vi "ゲージデータリセット.vi"(8 "測定周期/ms":dbl) -> (11 "実測設定項目配列_\nメインからの転記":T1[](array[typedef]) {"測定モード" items=["単発測定モード", "連続測定モード", "多点測定モード"]})   [LabVIEW 2021]
uses:
  <vilib>/Utility/config.llb/Read Key (U32).vi
  <vilib>/Utility/config.llb/Read Key (String).vi
  <vilib>/Utility/config.llb/Read Key (I32).vi
  <vilib>/Utility/config.llb/Read Key (Boolean).vi
  <vilib>/Utility/config.llb/NI_LVConfig.lvlib
panel:
  out "メイン設定_設定 12":T1 {"測定モード" items=["単発測定モード", "連続測定モード", "多点測定モード"]}
  out "メイン設定_設定 11":T1 {"測定モード" items=["単発測定モード", "連続測定モード", "多点測定モード"]}
  out "メイン設定_設定 10":T1 {"測定モード" items=["単発測定モード", "連続測定モード", "多点測定モード"]}
  out "メイン設定_設定 9":T1 {"測定モード" items=["単発測定モード", "連続測定モード", "多点測定モード"]}
  out "メイン設定_設定 8":T1 {"測定モード" items=["単発測定モード", "連続測定モード", "多点測定モード"]}
  out "メイン設定_設定 7":T1 {"測定モード" items=["単発測定モード", "連続測定モード", "多点測定モード"]}
  out "メイン設定_設定 6":T1 {"測定モード" items=["単発測定モード", "連続測定モード", "多点測定モード"]}
  out "メイン設定_設定 5":T1 {"測定モード" items=["単発測定モード", "連続測定モード", "多点測定モード"]}
  out "メイン設定_設定 4":T1 {"測定モード" items=["単発測定モード", "連続測定モード", "多点測定モード"]}
  out "メイン設定_設定 3":T1 {"測定モード" items=["単発測定モード", "連続測定モード", "多点測定モード"]}
  out "メイン設定_設定 2":T1 {"測定モード" items=["単発測定モード", "連続測定モード", "多点測定モード"]}
  out "メイン設定_設定 1":T1 {"測定モード" items=["単発測定モード", "連続測定モード", "多点測定モード"]}
  out "setup.iniエラーout":errorcluster caption="エラー入力（エラーなし）"
  out "iniフォルダパス取得":path
  in  "setup.iniエラーin":errorcluster caption="エラー入力（エラーなし）"
  out "ゲージエラー 12":errorcluster caption="エラー入力 (エラーなし)"
  out "ゲージエラー 11":errorcluster caption="エラー入力 (エラーなし)"
  out "ゲージエラー 10":errorcluster caption="エラー入力 (エラーなし)"
  out "ゲージエラー 9":errorcluster caption="エラー入力 (エラーなし)"
  out "ゲージエラー 8":errorcluster caption="エラー入力 (エラーなし)"
  out "ゲージエラー 7":errorcluster caption="エラー入力 (エラーなし)"
  out "ゲージエラー 6":errorcluster caption="エラー入力 (エラーなし)"
  out "ゲージエラー 5":errorcluster caption="エラー入力 (エラーなし)"
  out "ゲージエラー 4":errorcluster caption="エラー入力 (エラーなし)"
  out "ゲージエラー 3":errorcluster caption="エラー入力 (エラーなし)"
  out "ゲージエラー 2":errorcluster caption="エラー入力 (エラーなし)"
  out "ゲージエラー 1":errorcluster caption="エラー入力 (エラーなし)"
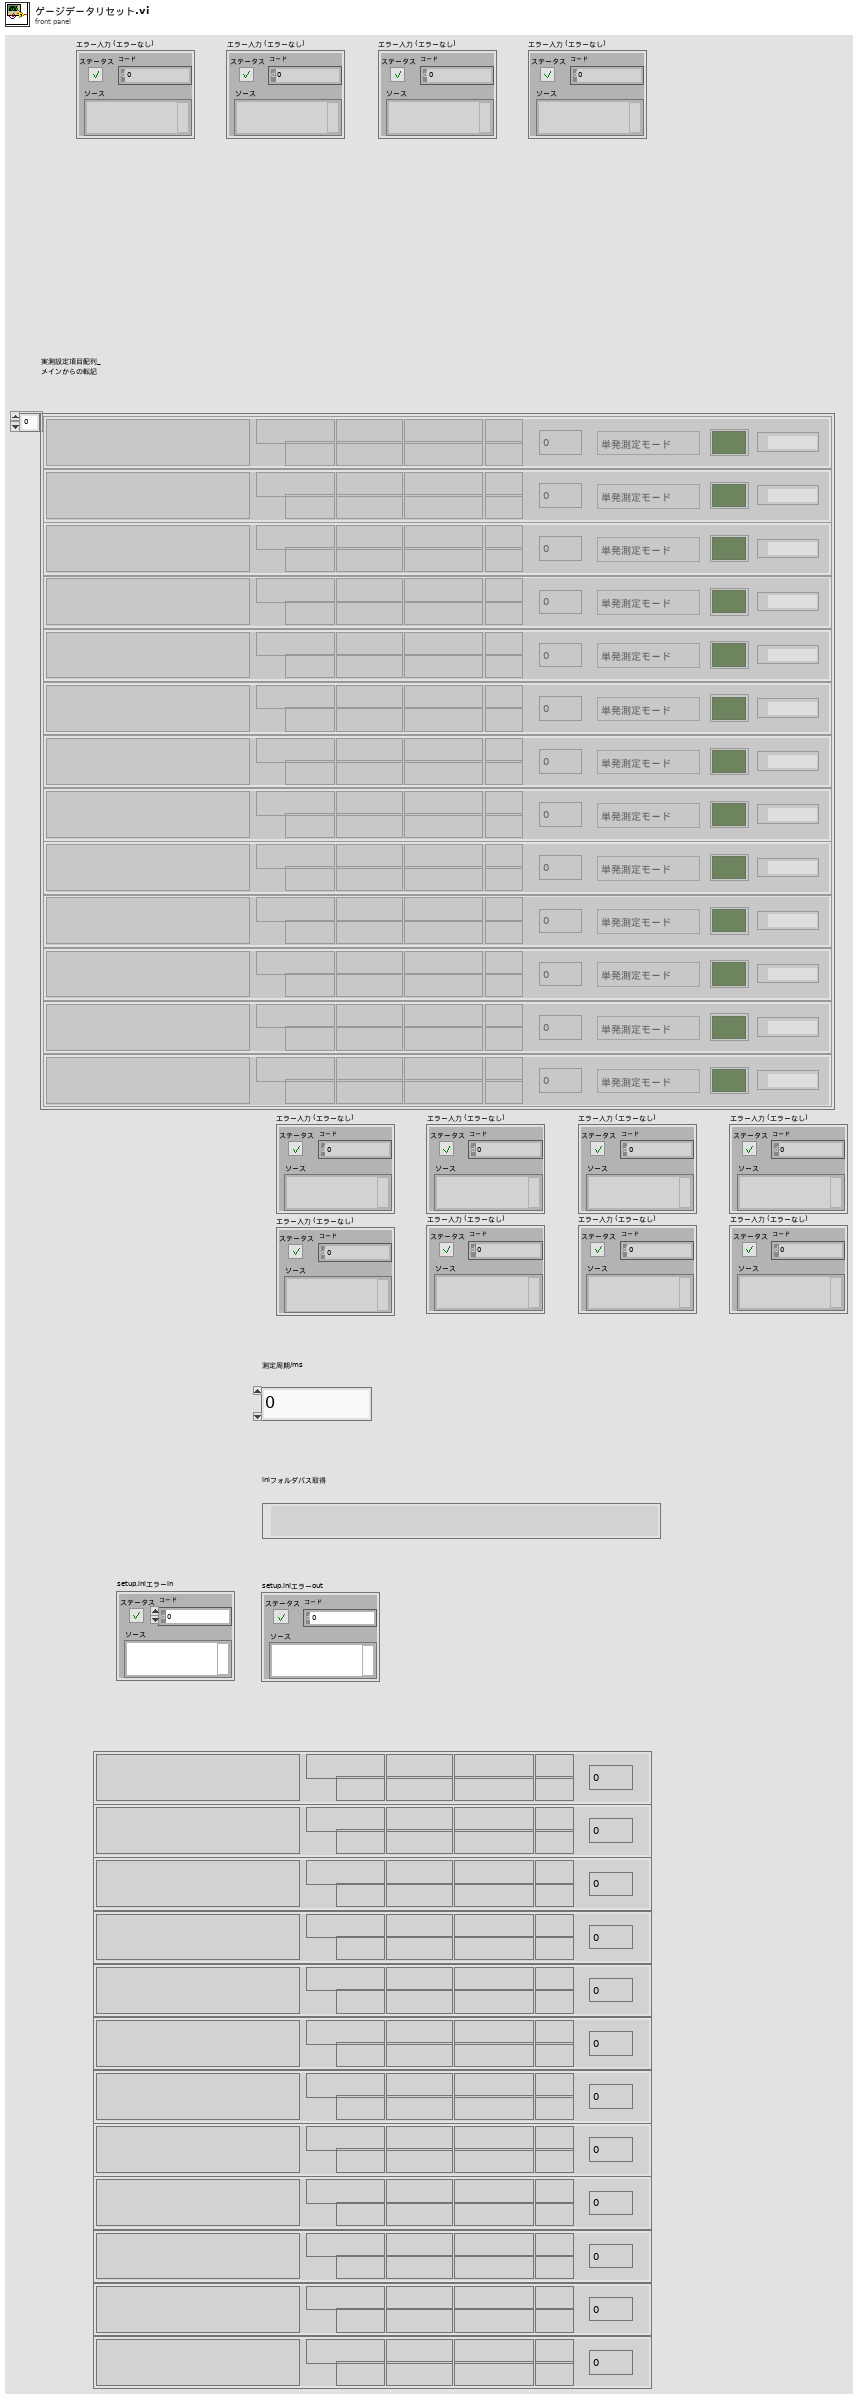
[diagram p1: front panel]
types:
  T1 = typedef "設定全項目制御器.ctl" = cluster{"規格":string, "規格上限":string, "規格下限":string, "ポートNo.":dbl, "測定モード":u16, "規格単位":string, "品質チェック項目":string, "測定周期":dbl, "実測値MAX":string, "実測値MIN":string, "実測値(MAX)":string, "実測値(MIN)":string, "測定画面表示ボタン":bool, "ゲージポートNo":refnum<visa-resource-name>}
  T2 = typedef "NI_LVConfig.lvlib/Config Data RefNum.ctl" = refnum<k1>
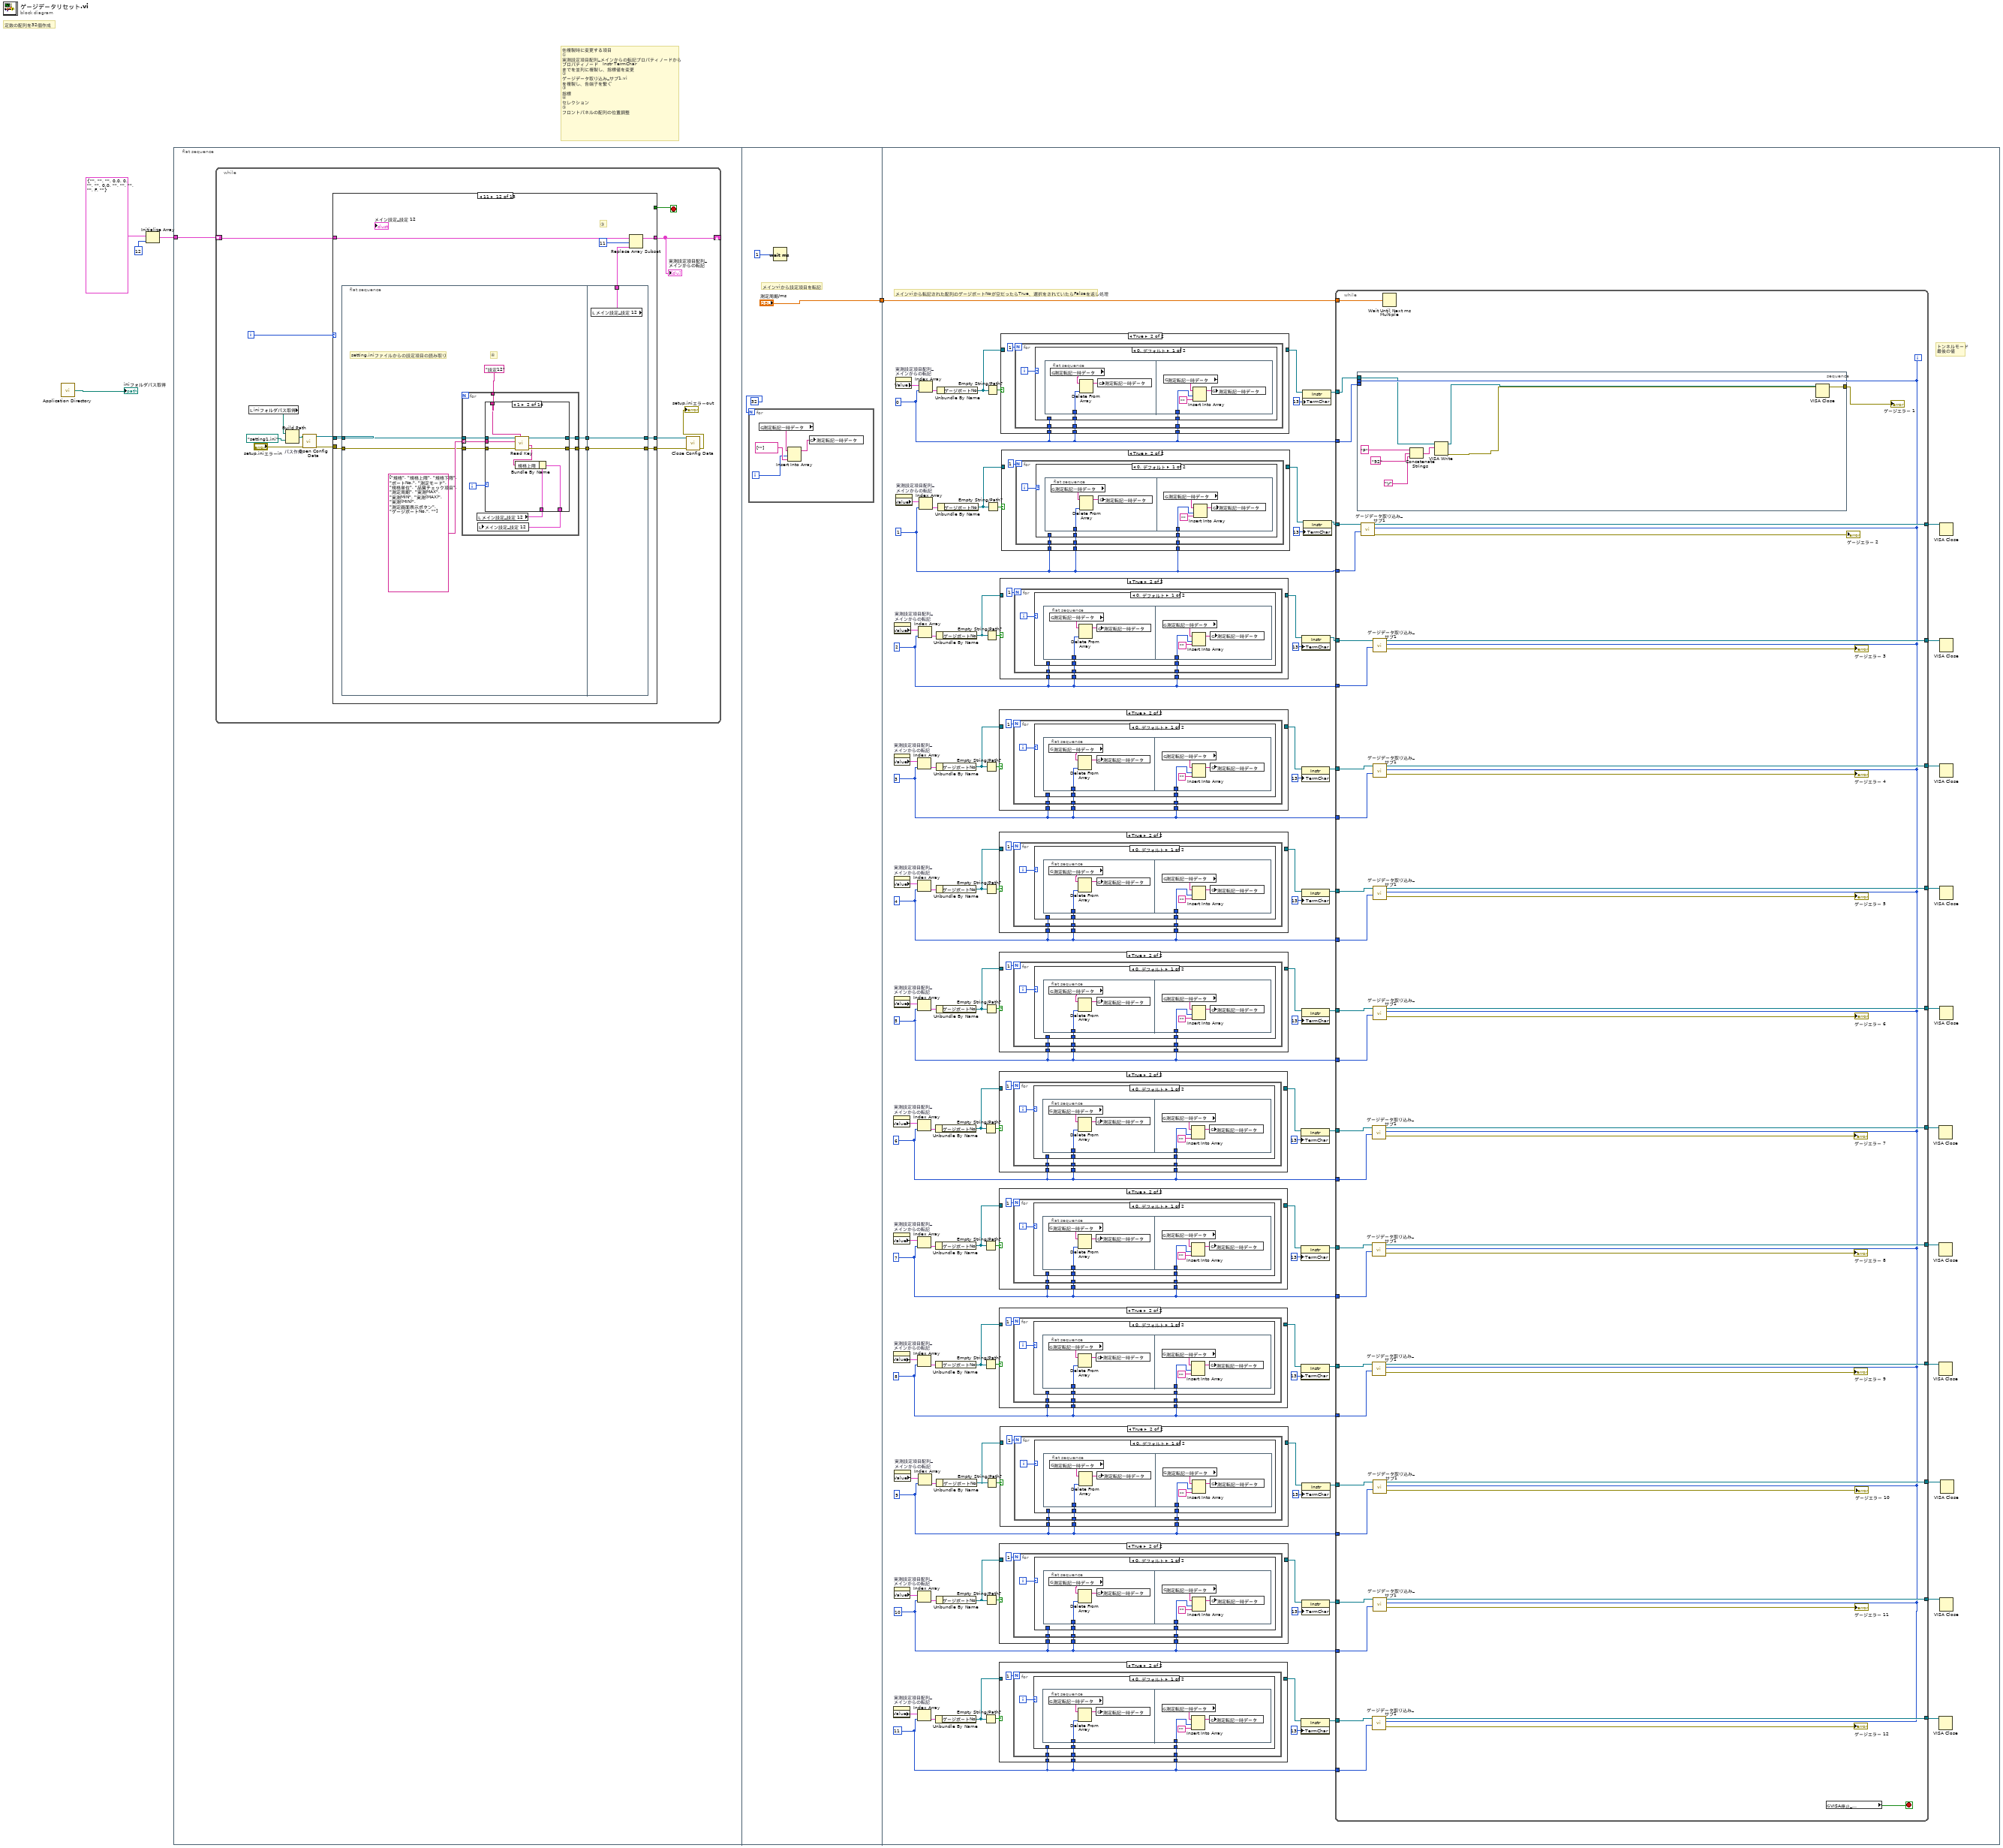
[diagram p0: block diagram]
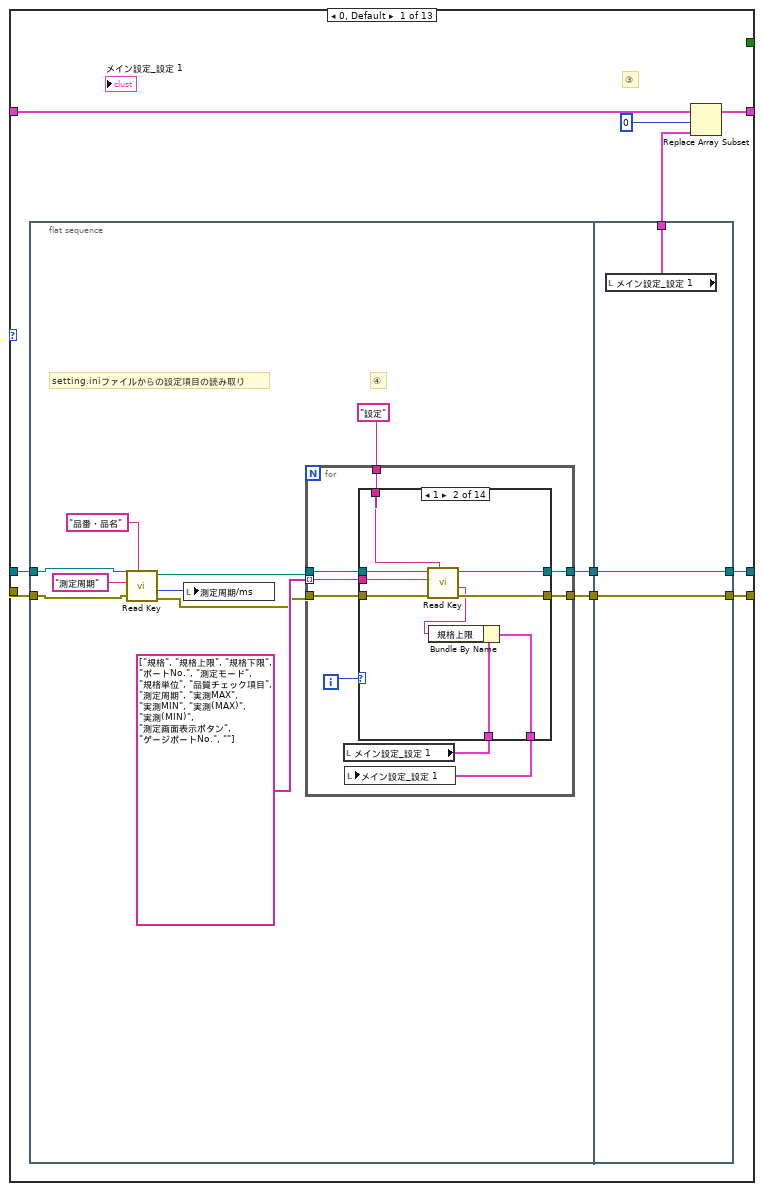
[diagram p2: hidden frame]
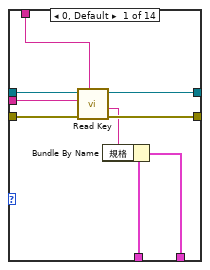
[diagram p3: hidden frame]
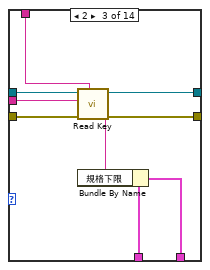
[diagram p4: hidden frame]
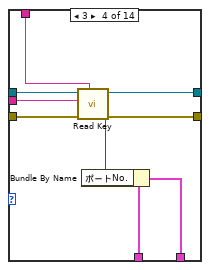
[diagram p5: hidden frame]
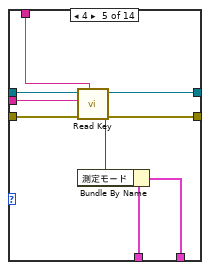
[diagram p6: hidden frame]
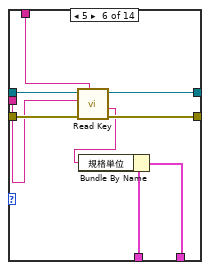
[diagram p7: hidden frame]
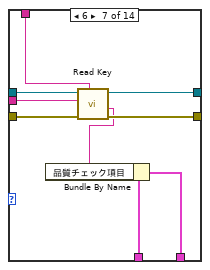
[diagram p8: hidden frame]
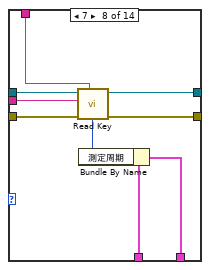
[diagram p9: hidden frame]
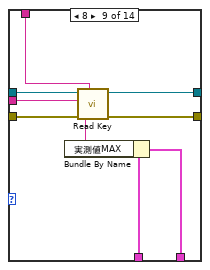
[diagram p10: hidden frame]
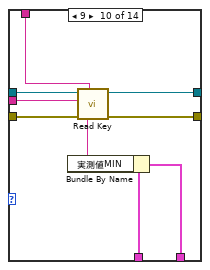
[diagram p11: hidden frame]
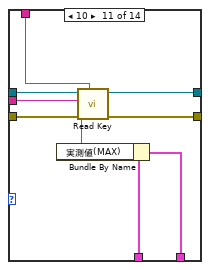
[diagram p12: hidden frame]
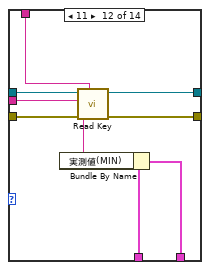
[diagram p13: hidden frame]
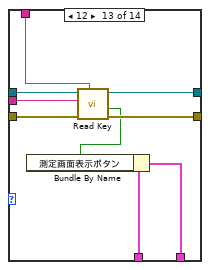
[diagram p14: hidden frame]
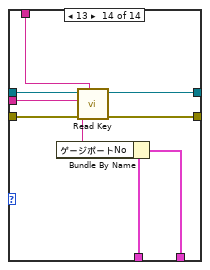
[diagram p15: hidden frame]
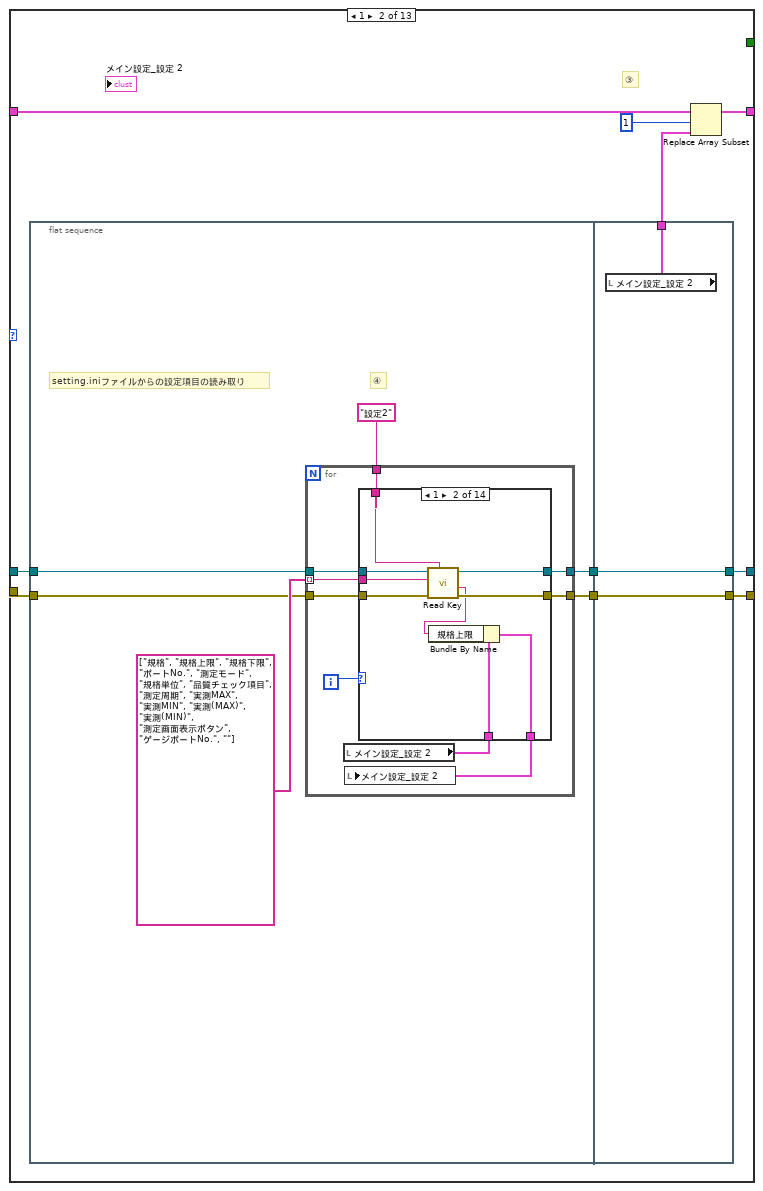
[diagram p16: hidden frame]
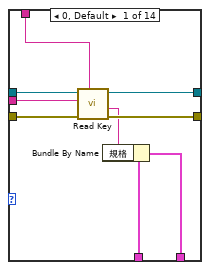
[diagram p17: hidden frame]
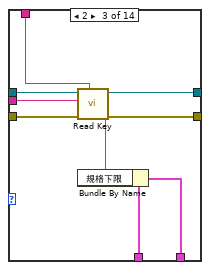
[diagram p18: hidden frame]
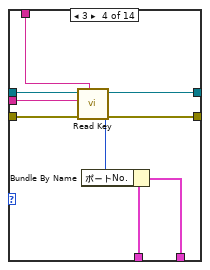
[diagram p19: hidden frame]
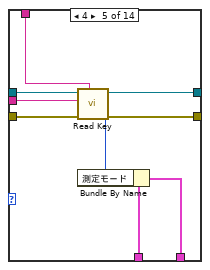
[diagram p20: hidden frame]
diagram:
  # "他複製時に変更する項目\n①\n実測設定項目配列_メインからの転記プロパティノードから\nプロパティノード　Instr TermChar\nまでを並列に複製し、指標値を変更\n②\nゲージデータ取り込み_サブ1.vi\nを複製し、各端子を繋ぐ\n③\n指標\n④\nセレクション\n⑤\nフロントパネルの配列の位置調整"
  # "定数の配列を32個作成"
  n1 = call <vilib>:"Application Directory.vi"() -> ("Application Directory"=→"iniフォルダパス取得":path)
  n2 = Initialize Array(T1 {"規格"="", "規格上限"="", "規格下限"="", "ポートNo."=0.0, "測定モード"=0, "規格単位"="", "品質チェック項目"="", "測定周期"=0.0, "実測値MAX"="", "実測値MIN"="", "実測値(MAX)"="", "実測値(MIN)"="", "測定画面表示ボタン"=FALSE, "ゲージポートNo"=""} ("メイン設定_設定"), 12) -> (w1:T1[])
  n3 = flat-sequence {
    tunnel: w1 -> [w6]
    tunnel: ["測定周期/ms"] -> w5
    tunnel: w5 -> [w1982]
    frame #0 {
      n4 = while {
        shift-right: [w7] -> _
        shift-left: w6 -> [w9]
        i -> [w14]
        stop <- w8 stop-if-true
        n5 = local read "iniフォルダパス取得"() -> (w19:path)
        n6 = Build Path "パス作成"(base path=w19, name or relative path=path "setting1.ini") -> (appended path=w18:path)
        n7 = call <vilib>:"Open Config Data.vi"("error in (no error)"="setup.iniエラーin", "configuration file path"=w18) -> ("error out"=w12:errorcluster, "refnum"=w13:T2)  [unwired: 1 in, 7 out]
        n8 = case shown="11" w14 {
          tunnel: w13 -> [w29 w188 w342 w496 w650 w804 w958 w1112 w1266 w1420 w1574 w1728 w1874]
          tunnel: w12 -> [w28 w187 w341 w495 w649 w803 w957 w1111 w1265 w1419 w1573 w1727 w1873]
          tunnel: [w27 w186 w340 w494 w648 w802 w956 w1110 w1264 w1418 w1572 w1726 w1874] -> w11
          tunnel: [w26 w185 w339 w493 w647 w801 w955 w1109 w1263 w1417 w1571 w1725 w1873] -> w10
          tunnel: w9 -> [w23 w182 w336 w490 w644 w798 w952 w1106 w1260 w1414 w1568 w1722 w1875]
          tunnel: [w22 w181 w335 w489 w643 w797 w951 w1105 w1259 w1413 w1567 w1721 w1875] -> w7
          tunnel: [_ _ _ _ _ _ _ _ _ _ _ _ TRUE] -> w8
          frame 0, Default {
            # "③"
            n9 = flat-sequence {
              tunnel: w29 -> [w33]
              tunnel: w28 -> [w31]
              tunnel: [w40] -> w25
              tunnel: [w39] -> w24
              tunnel: [w177] -> w26
              tunnel: [w178] -> w27
              tunnel: w25 -> [w178]
              tunnel: w24 -> [w177]
              tunnel: [w176] -> w21
              frame #0 {
                # "④"
                # "setting.iniファイルからの設定項目の読み取り"
                n10 = call-poly <vilib>:"Read Key.vi"("section"="品番・品名", "error in (no error)"=w31, "key"="測定周期", "refnum"=w33) -> ("error out"=w30:errorcluster, "value"=w35:u32, "refnum out"=w32:T2)  [unwired: 4 in, 1 out]
                n11 = local write "測定周期/ms"(w35) -> ()
                n12 = for {
                  tunnel: "設定" -> [w48]
                  tunnel: string[] ["規格", "規格上限", "規格下限", "ポートNo.", "測定モード", "規格単位", "品質チェック項目", "測定周期", "実測MAX", "実測MIN", "実測(MAX)", "実測(MIN)", "測定画面表示ボタン", "ゲージポートNo.", ""] -> [w43] mode=indexing
                  tunnel: w30 -> [w45]
                  tunnel: [w44] -> w39
                  tunnel: w32 -> [w49]
                  tunnel: [w47] -> w40
                  i -> [w46]
                  n13 = local read "メイン設定_設定 1"() -> (w41:T1)
                  n14 = case shown="1" w46 {
                    tunnel: w49 -> [w58 w67 w76 w85 w94 w103 w112 w121 w130 w139 w148 w157 w166 w175]
                    tunnel: [w57 w66 w75 w84 w93 w102 w111 w120 w129 w138 w147 w156 w165 w174] -> w47
                    tunnel: w48 -> [w56 w65 w74 w83 w92 w101 w110 w119 w128 w137 w146 w155 w164 w173]
                    tunnel: w45 -> [w55 w64 w73 w82 w91 w100 w109 w118 w127 w136 w145 w154 w163 w172]
                    tunnel: [w54 w63 w72 w81 w90 w99 w108 w117 w126 w135 w144 w153 w162 w171] -> w44
                    tunnel: w43 -> [w52 w61 w70 w79 w88 w97 w106 w115 w124 w133 w142 w151 w160 w169]
                    tunnel: [w51 w60 w69 w78 w87 w95 w104 w113 w123 w132 w141 w150 w159 w168] -> w42
                    tunnel: w41 -> [w50 w59 w68 w77 w86 w96 w105 w114 w122 w131 w140 w149 w158 w167]
                    frame 0, Default {
                      n15 = call-poly <vilib>:"Read Key.vi"("section"=w56, "error in (no error)"=w55, "key"=w52, "refnum"=w58) -> ("error out"=w54:errorcluster, "value"=w53:string, "refnum out"=w57:T2)  [unwired: 4 in, 1 out]
                      n16 = Bundle By Name(cluster=w50, "規格"=w53) -> (w51:T1)
                    }
                    frame 1 {
                      n17 = call-poly <vilib>:"Read Key.vi"("section"=w65, "error in (no error)"=w64, "key"=w61, "refnum"=w67) -> ("error out"=w63:errorcluster, "value"=w62:string, "refnum out"=w66:T2)  [unwired: 4 in, 1 out]
                      n18 = Bundle By Name(cluster=w59, "規格上限"=w62) -> (w60:T1)
                    }
                    frame 2 {
                      n19 = call-poly <vilib>:"Read Key.vi"("section"=w74, "error in (no error)"=w73, "key"=w70, "refnum"=w76) -> ("error out"=w72:errorcluster, "value"=w71:string, "refnum out"=w75:T2)  [unwired: 4 in, 1 out]
                      n20 = Bundle By Name(cluster=w68, "規格下限"=w71) -> (w69:T1)
                    }
                    frame 3 {
                      n21 = call-poly <vilib>:"Read Key.vi"("section"=w83, "error in (no error)"=w82, "key"=w79, "refnum"=w85) -> ("error out"=w81:errorcluster, "value"=w80:i32, "refnum out"=w84:T2)  [unwired: 4 in, 1 out]
                      n22 = Bundle By Name(cluster=w77, "ポートNo."=w80) -> (w78:T1)
                    }
                    frame 4 {
                      n23 = call-poly <vilib>:"Read Key.vi"("section"=w92, "error in (no error)"=w91, "key"=w88, "refnum"=w94) -> ("error out"=w90:errorcluster, "value"=w89:i32, "refnum out"=w93:T2)  [unwired: 4 in, 1 out]
                      n24 = Bundle By Name(cluster=w86, "測定モード"=w89) -> (w87:T1)
                    }
                    frame 5 {
                      n25 = call-poly <vilib>:"Read Key.vi"("section"=w101, "error in (no error)"=w100, "key"=w97, "refnum"=w103) -> ("error out"=w99:errorcluster, "value"=w98:string, "refnum out"=w102:T2)  [unwired: 4 in, 1 out]
                      n26 = Bundle By Name(cluster=w96, "規格単位"=w98) -> (w95:T1)
                    }
                    frame 6 {
                      n27 = call-poly <vilib>:"Read Key.vi"("section"=w110, "error in (no error)"=w109, "key"=w106, "refnum"=w112) -> ("error out"=w108:errorcluster, "value"=w107:string, "refnum out"=w111:T2)  [unwired: 4 in, 1 out]
                      n28 = Bundle By Name(cluster=w105, "品質チェック項目"=w107) -> (w104:T1)
                    }
                    frame 7 {
                      n29 = call-poly <vilib>:"Read Key.vi"("section"=w119, "error in (no error)"=w118, "key"=w115, "refnum"=w121) -> ("error out"=w117:errorcluster, "value"=w116:i32, "refnum out"=w120:T2)  [unwired: 4 in, 1 out]
                      n30 = Bundle By Name(cluster=w114, "測定周期"=w116) -> (w113:T1)
                    }
                    frame 8 {
                      n31 = call-poly <vilib>:"Read Key.vi"("section"=w128, "error in (no error)"=w127, "key"=w124, "refnum"=w130) -> ("error out"=w126:errorcluster, "value"=w125:string, "refnum out"=w129:T2)  [unwired: 4 in, 1 out]
                      n32 = Bundle By Name(cluster=w122, "実測値MAX"=w125) -> (w123:T1)
                    }
                    frame 9 {
                      n33 = call-poly <vilib>:"Read Key.vi"("section"=w137, "error in (no error)"=w136, "key"=w133, "refnum"=w139) -> ("error out"=w135:errorcluster, "value"=w134:string, "refnum out"=w138:T2)  [unwired: 4 in, 1 out]
                      n34 = Bundle By Name(cluster=w131, "実測値MIN"=w134) -> (w132:T1)
                    }
                    frame 10 {
                      n35 = call-poly <vilib>:"Read Key.vi"("section"=w146, "error in (no error)"=w145, "key"=w142, "refnum"=w148) -> ("error out"=w144:errorcluster, "value"=w143:string, "refnum out"=w147:T2)  [unwired: 4 in, 1 out]
                      n36 = Bundle By Name(cluster=w140, "実測値(MAX)"=w143) -> (w141:T1)
                    }
                    frame 11 {
                      n37 = call-poly <vilib>:"Read Key.vi"("section"=w155, "error in (no error)"=w154, "key"=w151, "refnum"=w157) -> ("error out"=w153:errorcluster, "value"=w152:string, "refnum out"=w156:T2)  [unwired: 4 in, 1 out]
                      n38 = Bundle By Name(cluster=w149, "実測値(MIN)"=w152) -> (w150:T1)
                    }
                    frame 12 {
                      n39 = call-poly <vilib>:"Read Key.vi"("section"=w164, "error in (no error)"=w163, "key"=w160, "refnum"=w166) -> ("error out"=w162:errorcluster, "value"=w161:bool, "refnum out"=w165:T2)  [unwired: 4 in, 1 out]
                      n40 = Bundle By Name(cluster=w158, "測定画面表示ボタン"=w161) -> (w159:T1)
                    }
                    frame 13 {
                      n41 = call-poly <vilib>:"Read Key.vi"("section"=w173, "error in (no error)"=w172, "key"=w169, "refnum"=w175) -> ("error out"=w171:errorcluster, "value"=w170:string, "refnum out"=w174:T2)  [unwired: 4 in, 1 out]
                      n42 = Bundle By Name(cluster=w167, "ゲージポートNo"=w170) -> (w168:T1)
                    }
                  }
                  n43 = local write "メイン設定_設定 1"(w42) -> ()
                }
              }
              frame #1 {
                n44 = local read "メイン設定_設定 1"() -> (w176:T1)
              }
            }
            n45 = Replace Array Subset(array=w23, new element=w21, index=0) -> (w22:T1[])
          }
          frame 1 {
            # "③"
            n46 = flat-sequence {
              tunnel: w188 -> [w190]
              tunnel: w187 -> [w189]
              tunnel: [w194] -> w184
              tunnel: [w193] -> w183
              tunnel: [w331] -> w185
              tunnel: [w332] -> w186
              tunnel: w184 -> [w332]
              tunnel: w183 -> [w331]
              tunnel: [w330] -> w180
              frame #0 {
                # "④"
                # "setting.iniファイルからの設定項目の読み取り"
                n47 = for {
                  tunnel: "設定2" -> [w202]
                  tunnel: string[] ["規格", "規格上限", "規格下限", "ポートNo.", "測定モード", "規格単位", "品質チェック項目", "測定周期", "実測MAX", "実測MIN", "実測(MAX)", "実測(MIN)", "測定画面表示ボタン", "ゲージポートNo.", ""] -> [w197] mode=indexing
                  tunnel: w189 -> [w199]
                  tunnel: [w198] -> w193
                  tunnel: w190 -> [w203]
                  tunnel: [w201] -> w194
                  i -> [w200]
                  n48 = local read "メイン設定_設定 2"() -> (w195:T1)
                  n49 = case shown="1" w200 {
                    tunnel: w203 -> [w212 w221 w230 w239 w248 w257 w266 w275 w284 w293 w302 w311 w320 w329]
                    tunnel: [w211 w220 w229 w238 w247 w256 w265 w274 w283 w292 w301 w310 w319 w328] -> w201
                    tunnel: w202 -> [w210 w219 w228 w237 w246 w255 w264 w273 w282 w291 w300 w309 w318 w327]
                    tunnel: w199 -> [w209 w218 w227 w236 w245 w254 w263 w272 w281 w290 w299 w308 w317 w326]
                    tunnel: [w208 w217 w226 w235 w244 w253 w262 w271 w280 w289 w298 w307 w316 w325] -> w198
                    tunnel: w197 -> [w206 w215 w224 w233 w242 w251 w260 w269 w278 w287 w296 w305 w314 w323]
                    tunnel: [w205 w214 w223 w232 w241 w249 w258 w267 w277 w286 w295 w304 w313 w322] -> w196
                    tunnel: w195 -> [w204 w213 w222 w231 w240 w250 w259 w268 w276 w285 w294 w303 w312 w321]
                    frame 0, Default {
                      n50 = call-poly <vilib>:"Read Key.vi"("section"=w210, "error in (no error)"=w209, "key"=w206, "refnum"=w212) -> ("error out"=w208:errorcluster, "value"=w207:string, "refnum out"=w211:T2)  [unwired: 4 in, 1 out]
                      n51 = Bundle By Name(cluster=w204, "規格"=w207) -> (w205:T1)
                    }
                    frame 1 {
                      n52 = call-poly <vilib>:"Read Key.vi"("section"=w219, "error in (no error)"=w218, "key"=w215, "refnum"=w221) -> ("error out"=w217:errorcluster, "value"=w216:string, "refnum out"=w220:T2)  [unwired: 4 in, 1 out]
                      n53 = Bundle By Name(cluster=w213, "規格上限"=w216) -> (w214:T1)
                    }
                    frame 2 {
                      n54 = call-poly <vilib>:"Read Key.vi"("section"=w228, "error in (no error)"=w227, "key"=w224, "refnum"=w230) -> ("error out"=w226:errorcluster, "value"=w225:string, "refnum out"=w229:T2)  [unwired: 4 in, 1 out]
                      n55 = Bundle By Name(cluster=w222, "規格下限"=w225) -> (w223:T1)
                    }
                    frame 3 {
                      n56 = call-poly <vilib>:"Read Key.vi"("section"=w237, "error in (no error)"=w236, "key"=w233, "refnum"=w239) -> ("error out"=w235:errorcluster, "value"=w234:i32, "refnum out"=w238:T2)  [unwired: 4 in, 1 out]
                      n57 = Bundle By Name(cluster=w231, "ポートNo."=w234) -> (w232:T1)
                    }
                    frame 4 {
                      n58 = call-poly <vilib>:"Read Key.vi"("section"=w246, "error in (no error)"=w245, "key"=w242, "refnum"=w248) -> ("error out"=w244:errorcluster, "value"=w243:i32, "refnum out"=w247:T2)  [unwired: 4 in, 1 out]
                      n59 = Bundle By Name(cluster=w240, "測定モード"=w243) -> (w241:T1)
                    }
                    frame 5 {
                      n60 = call-poly <vilib>:"Read Key.vi"("section"=w255, "error in (no error)"=w254, "key"=w251, "refnum"=w257) -> ("error out"=w253:errorcluster, "value"=w252:string, "refnum out"=w256:T2)  [unwired: 4 in, 1 out]
                      n61 = Bundle By Name(cluster=w250, "規格単位"=w252) -> (w249:T1)
                    }
                    frame 6 {
                      n62 = call-poly <vilib>:"Read Key.vi"("section"=w264, "error in (no error)"=w263, "key"=w260, "refnum"=w266) -> ("error out"=w262:errorcluster, "value"=w261:string, "refnum out"=w265:T2)  [unwired: 4 in, 1 out]
                      n63 = Bundle By Name(cluster=w259, "品質チェック項目"=w261) -> (w258:T1)
                    }
                    frame 7 {
                      n64 = call-poly <vilib>:"Read Key.vi"("section"=w273, "error in (no error)"=w272, "key"=w269, "refnum"=w275) -> ("error out"=w271:errorcluster, "value"=w270:i32, "refnum out"=w274:T2)  [unwired: 4 in, 1 out]
                      n65 = Bundle By Name(cluster=w268, "測定周期"=w270) -> (w267:T1)
                    }
                    frame 8 {
                      n66 = call-poly <vilib>:"Read Key.vi"("section"=w282, "error in (no error)"=w281, "key"=w278, "refnum"=w284) -> ("error out"=w280:errorcluster, "value"=w279:string, "refnum out"=w283:T2)  [unwired: 4 in, 1 out]
                      n67 = Bundle By Name(cluster=w276, "実測値MAX"=w279) -> (w277:T1)
                    }
                    frame 9 {
                      n68 = call-poly <vilib>:"Read Key.vi"("section"=w291, "error in (no error)"=w290, "key"=w287, "refnum"=w293) -> ("error out"=w289:errorcluster, "value"=w288:string, "refnum out"=w292:T2)  [unwired: 4 in, 1 out]
                      n69 = Bundle By Name(cluster=w285, "実測値MIN"=w288) -> (w286:T1)
                    }
                    frame 10 {
                      n70 = call-poly <vilib>:"Read Key.vi"("section"=w300, "error in (no error)"=w299, "key"=w296, "refnum"=w302) -> ("error out"=w298:errorcluster, "value"=w297:string, "refnum out"=w301:T2)  [unwired: 4 in, 1 out]
                      n71 = Bundle By Name(cluster=w294, "実測値(MAX)"=w297) -> (w295:T1)
                    }
                    frame 11 {
                      n72 = call-poly <vilib>:"Read Key.vi"("section"=w309, "error in (no error)"=w308, "key"=w305, "refnum"=w311) -> ("error out"=w307:errorcluster, "value"=w306:string, "refnum out"=w310:T2)  [unwired: 4 in, 1 out]
                      n73 = Bundle By Name(cluster=w303, "実測値(MIN)"=w306) -> (w304:T1)
                    }
                    frame 12 {
                      n74 = call-poly <vilib>:"Read Key.vi"("section"=w318, "error in (no error)"=w317, "key"=w314, "refnum"=w320) -> ("error out"=w316:errorcluster, "value"=w315:bool, "refnum out"=w319:T2)  [unwired: 4 in, 1 out]
                      n75 = Bundle By Name(cluster=w312, "測定画面表示ボタン"=w315) -> (w313:T1)
                    }
                    frame 13 {
                      n76 = call-poly <vilib>:"Read Key.vi"("section"=w327, "error in (no error)"=w326, "key"=w323, "refnum"=w329) -> ("error out"=w325:errorcluster, "value"=w324:string, "refnum out"=w328:T2)  [unwired: 4 in, 1 out]
                      n77 = Bundle By Name(cluster=w321, "ゲージポートNo"=w324) -> (w322:T1)
                    }
                  }
                  n78 = local write "メイン設定_設定 2"(w196) -> ()
                }
              }
              frame #1 {
                n79 = local read "メイン設定_設定 2"() -> (w330:T1)
              }
            }
            n80 = Replace Array Subset(array=w182, new element=w180, index=1) -> (w181:T1[])
          }
          frame 2 {
            # "③"
            n81 = flat-sequence {
              tunnel: w342 -> [w344]
              tunnel: w341 -> [w343]
              tunnel: [w348] -> w338
              tunnel: [w347] -> w337
              tunnel: [w485] -> w339
              tunnel: [w486] -> w340
              tunnel: w338 -> [w486]
              tunnel: w337 -> [w485]
              tunnel: [w484] -> w334
              frame #0 {
                # "④"
                # "setting.iniファイルからの設定項目の読み取り"
                n82 = for {
                  tunnel: "設定3" -> [w356]
                  tunnel: string[] ["規格", "規格上限", "規格下限", "ポートNo.", "測定モード", "規格単位", "品質チェック項目", "測定周期", "実測MAX", "実測MIN", "実測(MAX)", "実測(MIN)", "測定画面表示ボタン", "ゲージポートNo.", ""] -> [w351] mode=indexing
                  tunnel: w343 -> [w353]
                  tunnel: [w352] -> w347
                  tunnel: w344 -> [w357]
                  tunnel: [w355] -> w348
                  i -> [w354]
                  n83 = local read "メイン設定_設定 3"() -> (w349:T1)
                  n84 = case shown="1" w354 {
                    tunnel: w357 -> [w366 w375 w384 w393 w402 w411 w420 w429 w438 w447 w456 w465 w474 w483]
                    tunnel: [w365 w374 w383 w392 w401 w410 w419 w428 w437 w446 w455 w464 w473 w482] -> w355
                    tunnel: w356 -> [w364 w373 w382 w391 w400 w409 w418 w427 w436 w445 w454 w463 w472 w481]
                    tunnel: w353 -> [w363 w372 w381 w390 w399 w408 w417 w426 w435 w444 w453 w462 w471 w480]
                    tunnel: [w362 w371 w380 w389 w398 w407 w416 w425 w434 w443 w452 w461 w470 w479] -> w352
                    tunnel: w351 -> [w360 w369 w378 w387 w396 w405 w414 w423 w432 w441 w450 w459 w468 w477]
                    tunnel: [w359 w368 w377 w386 w395 w403 w412 w421 w431 w440 w449 w458 w467 w476] -> w350
                    tunnel: w349 -> [w358 w367 w376 w385 w394 w404 w413 w422 w430 w439 w448 w457 w466 w475]
                    frame 0, Default {
                      n85 = call-poly <vilib>:"Read Key.vi"("section"=w364, "error in (no error)"=w363, "key"=w360, "refnum"=w366) -> ("error out"=w362:errorcluster, "value"=w361:string, "refnum out"=w365:T2)  [unwired: 4 in, 1 out]
                      n86 = Bundle By Name(cluster=w358, "規格"=w361) -> (w359:T1)
                    }
                    frame 1 {
                      n87 = call-poly <vilib>:"Read Key.vi"("section"=w373, "error in (no error)"=w372, "key"=w369, "refnum"=w375) -> ("error out"=w371:errorcluster, "value"=w370:string, "refnum out"=w374:T2)  [unwired: 4 in, 1 out]
                      n88 = Bundle By Name(cluster=w367, "規格上限"=w370) -> (w368:T1)
                    }
                    frame 2 {
                      n89 = call-poly <vilib>:"Read Key.vi"("section"=w382, "error in (no error)"=w381, "key"=w378, "refnum"=w384) -> ("error out"=w380:errorcluster, "value"=w379:string, "refnum out"=w383:T2)  [unwired: 4 in, 1 out]
                      n90 = Bundle By Name(cluster=w376, "規格下限"=w379) -> (w377:T1)
                    }
                    frame 3 {
                      n91 = call-poly <vilib>:"Read Key.vi"("section"=w391, "error in (no error)"=w390, "key"=w387, "refnum"=w393) -> ("error out"=w389:errorcluster, "value"=w388:i32, "refnum out"=w392:T2)  [unwired: 4 in, 1 out]
                      n92 = Bundle By Name(cluster=w385, "ポートNo."=w388) -> (w386:T1)
                    }
                    frame 4 {
                      n93 = call-poly <vilib>:"Read Key.vi"("section"=w400, "error in (no error)"=w399, "key"=w396, "refnum"=w402) -> ("error out"=w398:errorcluster, "value"=w397:i32, "refnum out"=w401:T2)  [unwired: 4 in, 1 out]
                      n94 = Bundle By Name(cluster=w394, "測定モード"=w397) -> (w395:T1)
                    }
                    frame 5 {
                      n95 = call-poly <vilib>:"Read Key.vi"("section"=w409, "error in (no error)"=w408, "key"=w405, "refnum"=w411) -> ("error out"=w407:errorcluster, "value"=w406:string, "refnum out"=w410:T2)  [unwired: 4 in, 1 out]
                      n96 = Bundle By Name(cluster=w404, "規格単位"=w406) -> (w403:T1)
                    }
                    frame 6 {
                      n97 = call-poly <vilib>:"Read Key.vi"("section"=w418, "error in (no error)"=w417, "key"=w414, "refnum"=w420) -> ("error out"=w416:errorcluster, "value"=w415:string, "refnum out"=w419:T2)  [unwired: 4 in, 1 out]
                      n98 = Bundle By Name(cluster=w413, "品質チェック項目"=w415) -> (w412:T1)
                    }
                    frame 7 {
                      n99 = call-poly <vilib>:"Read Key.vi"("section"=w427, "error in (no error)"=w426, "key"=w423, "refnum"=w429) -> ("error out"=w425:errorcluster, "value"=w424:i32, "refnum out"=w428:T2)  [unwired: 4 in, 1 out]
                      n100 = Bundle By Name(cluster=w422, "測定周期"=w424) -> (w421:T1)
                    }
                    frame 8 {
                      n101 = call-poly <vilib>:"Read Key.vi"("section"=w436, "error in (no error)"=w435, "key"=w432, "refnum"=w438) -> ("error out"=w434:errorcluster, "value"=w433:string, "refnum out"=w437:T2)  [unwired: 4 in, 1 out]
                      n102 = Bundle By Name(cluster=w430, "実測値MAX"=w433) -> (w431:T1)
                    }
                    frame 9 {
                      n103 = call-poly <vilib>:"Read Key.vi"("section"=w445, "error in (no error)"=w444, "key"=w441, "refnum"=w447) -> ("error out"=w443:errorcluster, "value"=w442:string, "refnum out"=w446:T2)  [unwired: 4 in, 1 out]
                      n104 = Bundle By Name(cluster=w439, "実測値MIN"=w442) -> (w440:T1)
                    }
                    frame 10 {
                      n105 = call-poly <vilib>:"Read Key.vi"("section"=w454, "error in (no error)"=w453, "key"=w450, "refnum"=w456) -> ("error out"=w452:errorcluster, "value"=w451:string, "refnum out"=w455:T2)  [unwired: 4 in, 1 out]
                      n106 = Bundle By Name(cluster=w448, "実測値(MAX)"=w451) -> (w449:T1)
                    }
                    frame 11 {
                      n107 = call-poly <vilib>:"Read Key.vi"("section"=w463, "error in (no error)"=w462, "key"=w459, "refnum"=w465) -> ("error out"=w461:errorcluster, "value"=w460:string, "refnum out"=w464:T2)  [unwired: 4 in, 1 out]
                      n108 = Bundle By Name(cluster=w457, "実測値(MIN)"=w460) -> (w458:T1)
                    }
                    frame 12 {
                      n109 = call-poly <vilib>:"Read Key.vi"("section"=w472, "error in (no error)"=w471, "key"=w468, "refnum"=w474) -> ("error out"=w470:errorcluster, "value"=w469:bool, "refnum out"=w473:T2)  [unwired: 4 in, 1 out]
                      n110 = Bundle By Name(cluster=w466, "測定画面表示ボタン"=w469) -> (w467:T1)
                    }
                    frame 13 {
                      n111 = call-poly <vilib>:"Read Key.vi"("section"=w481, "error in (no error)"=w480, "key"=w477, "refnum"=w483) -> ("error out"=w479:errorcluster, "value"=w478:string, "refnum out"=w482:T2)  [unwired: 4 in, 1 out]
                      n112 = Bundle By Name(cluster=w475, "ゲージポートNo"=w478) -> (w476:T1)
                    }
                  }
                  n113 = local write "メイン設定_設定 3"(w350) -> ()
                }
              }
              frame #1 {
                n114 = local read "メイン設定_設定 3"() -> (w484:T1)
              }
            }
            n115 = Replace Array Subset(array=w336, new element=w334, index=2) -> (w335:T1[])
          }
          frame 3 {
            # "③"
            n116 = flat-sequence {
              tunnel: w496 -> [w498]
              tunnel: w495 -> [w497]
              tunnel: [w502] -> w492
              tunnel: [w501] -> w491
              tunnel: [w639] -> w493
              tunnel: [w640] -> w494
              tunnel: w492 -> [w640]
              tunnel: w491 -> [w639]
              tunnel: [w638] -> w488
              frame #0 {
                # "④"
                # "setting.iniファイルからの設定項目の読み取り"
                n117 = for {
                  tunnel: "設定4" -> [w510]
                  tunnel: string[] ["規格", "規格上限", "規格下限", "ポートNo.", "測定モード", "規格単位", "品質チェック項目", "測定周期", "実測MAX", "実測MIN", "実測(MAX)", "実測(MIN)", "測定画面表示ボタン", "ゲージポートNo.", ""] -> [w505] mode=indexing
                  tunnel: w497 -> [w507]
                  tunnel: [w506] -> w501
                  tunnel: w498 -> [w511]
                  tunnel: [w509] -> w502
                  i -> [w508]
                  n118 = local read "メイン設定_設定 4"() -> (w503:T1)
                  n119 = case shown="1" w508 {
                    tunnel: w511 -> [w520 w529 w538 w547 w556 w565 w574 w583 w592 w601 w610 w619 w628 w637]
                    tunnel: [w519 w528 w537 w546 w555 w564 w573 w582 w591 w600 w609 w618 w627 w636] -> w509
                    tunnel: w510 -> [w518 w527 w536 w545 w554 w563 w572 w581 w590 w599 w608 w617 w626 w635]
                    tunnel: w507 -> [w517 w526 w535 w544 w553 w562 w571 w580 w589 w598 w607 w616 w625 w634]
                    tunnel: [w516 w525 w534 w543 w552 w561 w570 w579 w588 w597 w606 w615 w624 w633] -> w506
                    tunnel: w505 -> [w514 w523 w532 w541 w550 w559 w568 w577 w586 w595 w604 w613 w622 w631]
                    tunnel: [w513 w522 w531 w540 w549 w557 w566 w575 w585 w594 w603 w612 w621 w630] -> w504
                    tunnel: w503 -> [w512 w521 w530 w539 w548 w558 w567 w576 w584 w593 w602 w611 w620 w629]
                    frame 0, Default {
                      n120 = call-poly <vilib>:"Read Key.vi"("section"=w518, "error in (no error)"=w517, "key"=w514, "refnum"=w520) -> ("error out"=w516:errorcluster, "value"=w515:string, "refnum out"=w519:T2)  [unwired: 4 in, 1 out]
                      n121 = Bundle By Name(cluster=w512, "規格"=w515) -> (w513:T1)
                    }
                    frame 1 {
                      n122 = call-poly <vilib>:"Read Key.vi"("section"=w527, "error in (no error)"=w526, "key"=w523, "refnum"=w529) -> ("error out"=w525:errorcluster, "value"=w524:string, "refnum out"=w528:T2)  [unwired: 4 in, 1 out]
                      n123 = Bundle By Name(cluster=w521, "規格上限"=w524) -> (w522:T1)
                    }
                    frame 2 {
                      n124 = call-poly <vilib>:"Read Key.vi"("section"=w536, "error in (no error)"=w535, "key"=w532, "refnum"=w538) -> ("error out"=w534:errorcluster, "value"=w533:string, "refnum out"=w537:T2)  [unwired: 4 in, 1 out]
                      n125 = Bundle By Name(cluster=w530, "規格下限"=w533) -> (w531:T1)
                    }
                    frame 3 {
                      n126 = call-poly <vilib>:"Read Key.vi"("section"=w545, "error in (no error)"=w544, "key"=w541, "refnum"=w547) -> ("error out"=w543:errorcluster, "value"=w542:i32, "refnum out"=w546:T2)  [unwired: 4 in, 1 out]
                      n127 = Bundle By Name(cluster=w539, "ポートNo."=w542) -> (w540:T1)
                    }
                    frame 4 {
                      n128 = call-poly <vilib>:"Read Key.vi"("section"=w554, "error in (no error)"=w553, "key"=w550, "refnum"=w556) -> ("error out"=w552:errorcluster, "value"=w551:i32, "refnum out"=w555:T2)  [unwired: 4 in, 1 out]
                      n129 = Bundle By Name(cluster=w548, "測定モード"=w551) -> (w549:T1)
                    }
                    frame 5 {
                      n130 = call-poly <vilib>:"Read Key.vi"("section"=w563, "error in (no error)"=w562, "key"=w559, "refnum"=w565) -> ("error out"=w561:errorcluster, "value"=w560:string, "refnum out"=w564:T2)  [unwired: 4 in, 1 out]
                      n131 = Bundle By Name(cluster=w558, "規格単位"=w560) -> (w557:T1)
                    }
                    frame 6 {
                      n132 = call-poly <vilib>:"Read Key.vi"("section"=w572, "error in (no error)"=w571, "key"=w568, "refnum"=w574) -> ("error out"=w570:errorcluster, "value"=w569:string, "refnum out"=w573:T2)  [unwired: 4 in, 1 out]
                      n133 = Bundle By Name(cluster=w567, "品質チェック項目"=w569) -> (w566:T1)
                    }
                    frame 7 {
                      n134 = call-poly <vilib>:"Read Key.vi"("section"=w581, "error in (no error)"=w580, "key"=w577, "refnum"=w583) -> ("error out"=w579:errorcluster, "value"=w578:i32, "refnum out"=w582:T2)  [unwired: 4 in, 1 out]
                      n135 = Bundle By Name(cluster=w576, "測定周期"=w578) -> (w575:T1)
                    }
                    frame 8 {
                      n136 = call-poly <vilib>:"Read Key.vi"("section"=w590, "error in (no error)"=w589, "key"=w586, "refnum"=w592) -> ("error out"=w588:errorcluster, "value"=w587:string, "refnum out"=w591:T2)  [unwired: 4 in, 1 out]
                      n137 = Bundle By Name(cluster=w584, "実測値MAX"=w587) -> (w585:T1)
                    }
                    frame 9 {
                      n138 = call-poly <vilib>:"Read Key.vi"("section"=w599, "error in (no error)"=w598, "key"=w595, "refnum"=w601) -> ("error out"=w597:errorcluster, "value"=w596:string, "refnum out"=w600:T2)  [unwired: 4 in, 1 out]
                      n139 = Bundle By Name(cluster=w593, "実測値MIN"=w596) -> (w594:T1)
                    }
                    frame 10 {
                      n140 = call-poly <vilib>:"Read Key.vi"("section"=w608, "error in (no error)"=w607, "key"=w604, "refnum"=w610) -> ("error out"=w606:errorcluster, "value"=w605:string, "refnum out"=w609:T2)  [unwired: 4 in, 1 out]
                      n141 = Bundle By Name(cluster=w602, "実測値(MAX)"=w605) -> (w603:T1)
                    }
                    frame 11 {
                      n142 = call-poly <vilib>:"Read Key.vi"("section"=w617, "error in (no error)"=w616, "key"=w613, "refnum"=w619) -> ("error out"=w615:errorcluster, "value"=w614:string, "refnum out"=w618:T2)  [unwired: 4 in, 1 out]
                      n143 = Bundle By Name(cluster=w611, "実測値(MIN)"=w614) -> (w612:T1)
                    }
                    frame 12 {
                      n144 = call-poly <vilib>:"Read Key.vi"("section"=w626, "error in (no error)"=w625, "key"=w622, "refnum"=w628) -> ("error out"=w624:errorcluster, "value"=w623:bool, "refnum out"=w627:T2)  [unwired: 4 in, 1 out]
                      n145 = Bundle By Name(cluster=w620, "測定画面表示ボタン"=w623) -> (w621:T1)
                    }
                    frame 13 {
                      n146 = call-poly <vilib>:"Read Key.vi"("section"=w635, "error in (no error)"=w634, "key"=w631, "refnum"=w637) -> ("error out"=w633:errorcluster, "value"=w632:string, "refnum out"=w636:T2)  [unwired: 4 in, 1 out]
                      n147 = Bundle By Name(cluster=w629, "ゲージポートNo"=w632) -> (w630:T1)
                    }
                  }
                  n148 = local write "メイン設定_設定 4"(w504) -> ()
                }
              }
              frame #1 {
                n149 = local read "メイン設定_設定 4"() -> (w638:T1)
              }
            }
            n150 = Replace Array Subset(array=w490, new element=w488, index=3) -> (w489:T1[])
          }
          frame 4 {
            # "③"
            n151 = flat-sequence {
              tunnel: w650 -> [w652]
              tunnel: w649 -> [w651]
              tunnel: [w656] -> w646
              tunnel: [w655] -> w645
              tunnel: [w793] -> w647
              tunnel: [w794] -> w648
              tunnel: w646 -> [w794]
              tunnel: w645 -> [w793]
              tunnel: [w792] -> w642
              frame #0 {
                # "④"
                # "setting.iniファイルからの設定項目の読み取り"
                n152 = for {
                  tunnel: "設定5" -> [w664]
                  tunnel: string[] ["規格", "規格上限", "規格下限", "ポートNo.", "測定モード", "規格単位", "品質チェック項目", "測定周期", "実測MAX", "実測MIN", "実測(MAX)", "実測(MIN)", "測定画面表示ボタン", "ゲージポートNo.", ""] -> [w659] mode=indexing
                  tunnel: w651 -> [w661]
                  tunnel: [w660] -> w655
                  tunnel: w652 -> [w665]
                  tunnel: [w663] -> w656
                  i -> [w662]
                  n153 = local read "メイン設定_設定 5"() -> (w657:T1)
                  n154 = case shown="1" w662 {
                    tunnel: w665 -> [w674 w683 w692 w701 w710 w719 w728 w737 w746 w755 w764 w773 w782 w791]
                    tunnel: [w673 w682 w691 w700 w709 w718 w727 w736 w745 w754 w763 w772 w781 w790] -> w663
                    tunnel: w664 -> [w672 w681 w690 w699 w708 w717 w726 w735 w744 w753 w762 w771 w780 w789]
                    tunnel: w661 -> [w671 w680 w689 w698 w707 w716 w725 w734 w743 w752 w761 w770 w779 w788]
                    tunnel: [w670 w679 w688 w697 w706 w715 w724 w733 w742 w751 w760 w769 w778 w787] -> w660
                    tunnel: w659 -> [w668 w677 w686 w695 w704 w713 w722 w731 w740 w749 w758 w767 w776 w785]
                    tunnel: [w667 w676 w685 w694 w703 w711 w720 w729 w739 w748 w757 w766 w775 w784] -> w658
                    tunnel: w657 -> [w666 w675 w684 w693 w702 w712 w721 w730 w738 w747 w756 w765 w774 w783]
                    frame 0, Default {
                      n155 = call-poly <vilib>:"Read Key.vi"("section"=w672, "error in (no error)"=w671, "key"=w668, "refnum"=w674) -> ("error out"=w670:errorcluster, "value"=w669:string, "refnum out"=w673:T2)  [unwired: 4 in, 1 out]
                      n156 = Bundle By Name(cluster=w666, "規格"=w669) -> (w667:T1)
                    }
                    frame 1 {
                      n157 = call-poly <vilib>:"Read Key.vi"("section"=w681, "error in (no error)"=w680, "key"=w677, "refnum"=w683) -> ("error out"=w679:errorcluster, "value"=w678:string, "refnum out"=w682:T2)  [unwired: 4 in, 1 out]
                      n158 = Bundle By Name(cluster=w675, "規格上限"=w678) -> (w676:T1)
                    }
                    frame 2 {
                      n159 = call-poly <vilib>:"Read Key.vi"("section"=w690, "error in (no error)"=w689, "key"=w686, "refnum"=w692) -> ("error out"=w688:errorcluster, "value"=w687:string, "refnum out"=w691:T2)  [unwired: 4 in, 1 out]
                      n160 = Bundle By Name(cluster=w684, "規格下限"=w687) -> (w685:T1)
                    }
                    frame 3 {
                      n161 = call-poly <vilib>:"Read Key.vi"("section"=w699, "error in (no error)"=w698, "key"=w695, "refnum"=w701) -> ("error out"=w697:errorcluster, "value"=w696:i32, "refnum out"=w700:T2)  [unwired: 4 in, 1 out]
                      n162 = Bundle By Name(cluster=w693, "ポートNo."=w696) -> (w694:T1)
                    }
                    frame 4 {
                      n163 = call-poly <vilib>:"Read Key.vi"("section"=w708, "error in (no error)"=w707, "key"=w704, "refnum"=w710) -> ("error out"=w706:errorcluster, "value"=w705:i32, "refnum out"=w709:T2)  [unwired: 4 in, 1 out]
                      n164 = Bundle By Name(cluster=w702, "測定モード"=w705) -> (w703:T1)
                    }
                    frame 5 {
                      n165 = call-poly <vilib>:"Read Key.vi"("section"=w717, "error in (no error)"=w716, "key"=w713, "refnum"=w719) -> ("error out"=w715:errorcluster, "value"=w714:string, "refnum out"=w718:T2)  [unwired: 4 in, 1 out]
                      n166 = Bundle By Name(cluster=w712, "規格単位"=w714) -> (w711:T1)
                    }
                    frame 6 {
                      n167 = call-poly <vilib>:"Read Key.vi"("section"=w726, "error in (no error)"=w725, "key"=w722, "refnum"=w728) -> ("error out"=w724:errorcluster, "value"=w723:string, "refnum out"=w727:T2)  [unwired: 4 in, 1 out]
                      n168 = Bundle By Name(cluster=w721, "品質チェック項目"=w723) -> (w720:T1)
                    }
                    frame 7 {
                      n169 = call-poly <vilib>:"Read Key.vi"("section"=w735, "error in (no error)"=w734, "key"=w731, "refnum"=w737) -> ("error out"=w733:errorcluster, "value"=w732:i32, "refnum out"=w736:T2)  [unwired: 4 in, 1 out]
                      n170 = Bundle By Name(cluster=w730, "測定周期"=w732) -> (w729:T1)
                    }
                    frame 8 {
                      n171 = call-poly <vilib>:"Read Key.vi"("section"=w744, "error in (no error)"=w743, "key"=w740, "refnum"=w746) -> ("error out"=w742:errorcluster, "value"=w741:string, "refnum out"=w745:T2)  [unwired: 4 in, 1 out]
                      n172 = Bundle By Name(cluster=w738, "実測値MAX"=w741) -> (w739:T1)
                    }
                    frame 9 {
                      n173 = call-poly <vilib>:"Read Key.vi"("section"=w753, "error in (no error)"=w752, "key"=w749, "refnum"=w755) -> ("error out"=w751:errorcluster, "value"=w750:string, "refnum out"=w754:T2)  [unwired: 4 in, 1 out]
                      n174 = Bundle By Name(cluster=w747, "実測値MIN"=w750) -> (w748:T1)
                    }
                    frame 10 {
                      n175 = call-poly <vilib>:"Read Key.vi"("section"=w762, "error in (no error)"=w761, "key"=w758, "refnum"=w764) -> ("error out"=w760:errorcluster, "value"=w759:string, "refnum out"=w763:T2)  [unwired: 4 in, 1 out]
                      n176 = Bundle By Name(cluster=w756, "実測値(MAX)"=w759) -> (w757:T1)
                    }
                    frame 11 {
                      n177 = call-poly <vilib>:"Read Key.vi"("section"=w771, "error in (no error)"=w770, "key"=w767, "refnum"=w773) -> ("error out"=w769:errorcluster, "value"=w768:string, "refnum out"=w772:T2)  [unwired: 4 in, 1 out]
                      n178 = Bundle By Name(cluster=w765, "実測値(MIN)"=w768) -> (w766:T1)
                    }
                    frame 12 {
                      n179 = call-poly <vilib>:"Read Key.vi"("section"=w780, "error in (no error)"=w779, "key"=w776, "refnum"=w782) -> ("error out"=w778:errorcluster, "value"=w777:bool, "refnum out"=w781:T2)  [unwired: 4 in, 1 out]
                      n180 = Bundle By Name(cluster=w774, "測定画面表示ボタン"=w777) -> (w775:T1)
                    }
                    frame 13 {
                      n181 = call-poly <vilib>:"Read Key.vi"("section"=w789, "error in (no error)"=w788, "key"=w785, "refnum"=w791) -> ("error out"=w787:errorcluster, "value"=w786:string, "refnum out"=w790:T2)  [unwired: 4 in, 1 out]
                      n182 = Bundle By Name(cluster=w783, "ゲージポートNo"=w786) -> (w784:T1)
                    }
                  }
                  n183 = local write "メイン設定_設定 5"(w658) -> ()
                }
              }
              frame #1 {
                n184 = local read "メイン設定_設定 5"() -> (w792:T1)
              }
            }
            n185 = Replace Array Subset(array=w644, new element=w642, index=4) -> (w643:T1[])
          }
          frame 5 {
            # "③"
            n186 = flat-sequence {
              tunnel: w804 -> [w806]
              tunnel: w803 -> [w805]
              tunnel: [w810] -> w800
              tunnel: [w809] -> w799
              tunnel: [w947] -> w801
              tunnel: [w948] -> w802
              tunnel: w800 -> [w948]
              tunnel: w799 -> [w947]
              tunnel: [w946] -> w796
              frame #0 {
                # "④"
                # "setting.iniファイルからの設定項目の読み取り"
                n187 = for {
                  tunnel: "設定6" -> [w818]
                  tunnel: string[] ["規格", "規格上限", "規格下限", "ポートNo.", "測定モード", "規格単位", "品質チェック項目", "測定周期", "実測MAX", "実測MIN", "実測(MAX)", "実測(MIN)", "測定画面表示ボタン", "ゲージポートNo.", ""] -> [w813] mode=indexing
                  tunnel: w805 -> [w815]
                  tunnel: [w814] -> w809
                  tunnel: w806 -> [w819]
                  tunnel: [w817] -> w810
                  i -> [w816]
                  n188 = local read "メイン設定_設定 6"() -> (w811:T1)
                  n189 = case shown="1" w816 {
                    tunnel: w819 -> [w828 w837 w846 w855 w864 w873 w882 w891 w900 w909 w918 w927 w936 w945]
                    tunnel: [w827 w836 w845 w854 w863 w872 w881 w890 w899 w908 w917 w926 w935 w944] -> w817
                    tunnel: w818 -> [w826 w835 w844 w853 w862 w871 w880 w889 w898 w907 w916 w925 w934 w943]
                    tunnel: w815 -> [w825 w834 w843 w852 w861 w870 w879 w888 w897 w906 w915 w924 w933 w942]
                    tunnel: [w824 w833 w842 w851 w860 w869 w878 w887 w896 w905 w914 w923 w932 w941] -> w814
                    tunnel: w813 -> [w822 w831 w840 w849 w858 w867 w876 w885 w894 w903 w912 w921 w930 w939]
                    tunnel: [w821 w830 w839 w848 w857 w865 w874 w883 w893 w902 w911 w920 w929 w938] -> w812
                    tunnel: w811 -> [w820 w829 w838 w847 w856 w866 w875 w884 w892 w901 w910 w919 w928 w937]
                    frame 0, Default {
                      n190 = call-poly <vilib>:"Read Key.vi"("section"=w826, "error in (no error)"=w825, "key"=w822, "refnum"=w828) -> ("error out"=w824:errorcluster, "value"=w823:string, "refnum out"=w827:T2)  [unwired: 4 in, 1 out]
                      n191 = Bundle By Name(cluster=w820, "規格"=w823) -> (w821:T1)
                    }
                    frame 1 {
                      n192 = call-poly <vilib>:"Read Key.vi"("section"=w835, "error in (no error)"=w834, "key"=w831, "refnum"=w837) -> ("error out"=w833:errorcluster, "value"=w832:string, "refnum out"=w836:T2)  [unwired: 4 in, 1 out]
                      n193 = Bundle By Name(cluster=w829, "規格上限"=w832) -> (w830:T1)
                    }
                    frame 2 {
                      n194 = call-poly <vilib>:"Read Key.vi"("section"=w844, "error in (no error)"=w843, "key"=w840, "refnum"=w846) -> ("error out"=w842:errorcluster, "value"=w841:string, "refnum out"=w845:T2)  [unwired: 4 in, 1 out]
                      n195 = Bundle By Name(cluster=w838, "規格下限"=w841) -> (w839:T1)
                    }
                    frame 3 {
                      n196 = call-poly <vilib>:"Read Key.vi"("section"=w853, "error in (no error)"=w852, "key"=w849, "refnum"=w855) -> ("error out"=w851:errorcluster, "value"=w850:i32, "refnum out"=w854:T2)  [unwired: 4 in, 1 out]
                      n197 = Bundle By Name(cluster=w847, "ポートNo."=w850) -> (w848:T1)
                    }
                    frame 4 {
                      n198 = call-poly <vilib>:"Read Key.vi"("section"=w862, "error in (no error)"=w861, "key"=w858, "refnum"=w864) -> ("error out"=w860:errorcluster, "value"=w859:i32, "refnum out"=w863:T2)  [unwired: 4 in, 1 out]
                      n199 = Bundle By Name(cluster=w856, "測定モード"=w859) -> (w857:T1)
                    }
                    frame 5 {
                      n200 = call-poly <vilib>:"Read Key.vi"("section"=w871, "error in (no error)"=w870, "key"=w867, "refnum"=w873) -> ("error out"=w869:errorcluster, "value"=w868:string, "refnum out"=w872:T2)  [unwired: 4 in, 1 out]
                      n201 = Bundle By Name(cluster=w866, "規格単位"=w868) -> (w865:T1)
                    }
                    frame 6 {
                      n202 = call-poly <vilib>:"Read Key.vi"("section"=w880, "error in (no error)"=w879, "key"=w876, "refnum"=w882) -> ("error out"=w878:errorcluster, "value"=w877:string, "refnum out"=w881:T2)  [unwired: 4 in, 1 out]
                      n203 = Bundle By Name(cluster=w875, "品質チェック項目"=w877) -> (w874:T1)
                    }
                    frame 7 {
                      n204 = call-poly <vilib>:"Read Key.vi"("section"=w889, "error in (no error)"=w888, "key"=w885, "refnum"=w891) -> ("error out"=w887:errorcluster, "value"=w886:i32, "refnum out"=w890:T2)  [unwired: 4 in, 1 out]
                      n205 = Bundle By Name(cluster=w884, "測定周期"=w886) -> (w883:T1)
                    }
                    frame 8 {
                      n206 = call-poly <vilib>:"Read Key.vi"("section"=w898, "error in (no error)"=w897, "key"=w894, "refnum"=w900) -> ("error out"=w896:errorcluster, "value"=w895:string, "refnum out"=w899:T2)  [unwired: 4 in, 1 out]
                      n207 = Bundle By Name(cluster=w892, "実測値MAX"=w895) -> (w893:T1)
                    }
                    frame 9 {
                      n208 = call-poly <vilib>:"Read Key.vi"("section"=w907, "error in (no error)"=w906, "key"=w903, "refnum"=w909) -> ("error out"=w905:errorcluster, "value"=w904:string, "refnum out"=w908:T2)  [unwired: 4 in, 1 out]
                      n209 = Bundle By Name(cluster=w901, "実測値MIN"=w904) -> (w902:T1)
                    }
                    frame 10 {
                      n210 = call-poly <vilib>:"Read Key.vi"("section"=w916, "error in (no error)"=w915, "key"=w912, "refnum"=w918) -> ("error out"=w914:errorcluster, "value"=w913:string, "refnum out"=w917:T2)  [unwired: 4 in, 1 out]
                      n211 = Bundle By Name(cluster=w910, "実測値(MAX)"=w913) -> (w911:T1)
                    }
                    frame 11 {
                      n212 = call-poly <vilib>:"Read Key.vi"("section"=w925, "error in (no error)"=w924, "key"=w921, "refnum"=w927) -> ("error out"=w923:errorcluster, "value"=w922:string, "refnum out"=w926:T2)  [unwired: 4 in, 1 out]
                      n213 = Bundle By Name(cluster=w919, "実測値(MIN)"=w922) -> (w920:T1)
                    }
                    frame 12 {
                      n214 = call-poly <vilib>:"Read Key.vi"("section"=w934, "error in (no error)"=w933, "key"=w930, "refnum"=w936) -> ("error out"=w932:errorcluster, "value"=w931:bool, "refnum out"=w935:T2)  [unwired: 4 in, 1 out]
                      n215 = Bundle By Name(cluster=w928, "測定画面表示ボタン"=w931) -> (w929:T1)
                    }
                    frame 13 {
                      n216 = call-poly <vilib>:"Read Key.vi"("section"=w943, "error in (no error)"=w942, "key"=w939, "refnum"=w945) -> ("error out"=w941:errorcluster, "value"=w940:string, "refnum out"=w944:T2)  [unwired: 4 in, 1 out]
                      n217 = Bundle By Name(cluster=w937, "ゲージポートNo"=w940) -> (w938:T1)
                    }
                  }
                  n218 = local write "メイン設定_設定 6"(w812) -> ()
                }
              }
              frame #1 {
                n219 = local read "メイン設定_設定 6"() -> (w946:T1)
              }
            }
            n220 = Replace Array Subset(array=w798, new element=w796, index=5) -> (w797:T1[])
          }
          frame 6 {
            # "③"
            n221 = flat-sequence {
              tunnel: w958 -> [w960]
              tunnel: w957 -> [w959]
              tunnel: [w964] -> w954
              tunnel: [w963] -> w953
              tunnel: [w1101] -> w955
              tunnel: [w1102] -> w956
              tunnel: w954 -> [w1102]
              tunnel: w953 -> [w1101]
              tunnel: [w1100] -> w950
              frame #0 {
                # "④"
                # "setting.iniファイルからの設定項目の読み取り"
                n222 = for {
                  tunnel: "設定7" -> [w972]
                  tunnel: string[] ["規格", "規格上限", "規格下限", "ポートNo.", "測定モード", "規格単位", "品質チェック項目", "測定周期", "実測MAX", "実測MIN", "実測(MAX)", "実測(MIN)", "測定画面表示ボタン", "ゲージポートNo.", ""] -> [w967] mode=indexing
                  tunnel: w959 -> [w969]
                  tunnel: [w968] -> w963
                  tunnel: w960 -> [w973]
                  tunnel: [w971] -> w964
                  i -> [w970]
                  n223 = local read "メイン設定_設定 7"() -> (w965:T1)
                  n224 = case shown="1" w970 {
                    tunnel: w973 -> [w982 w991 w1000 w1009 w1018 w1027 w1036 w1045 w1054 w1063 w1072 w1081 w1090 w1099]
                    tunnel: [w981 w990 w999 w1008 w1017 w1026 w1035 w1044 w1053 w1062 w1071 w1080 w1089 w1098] -> w971
                    tunnel: w972 -> [w980 w989 w998 w1007 w1016 w1025 w1034 w1043 w1052 w1061 w1070 w1079 w1088 w1097]
                    tunnel: w969 -> [w979 w988 w997 w1006 w1015 w1024 w1033 w1042 w1051 w1060 w1069 w1078 w1087 w1096]
                    tunnel: [w978 w987 w996 w1005 w1014 w1023 w1032 w1041 w1050 w1059 w1068 w1077 w1086 w1095] -> w968
                    tunnel: w967 -> [w976 w985 w994 w1003 w1012 w1021 w1030 w1039 w1048 w1057 w1066 w1075 w1084 w1093]
                    tunnel: [w975 w984 w993 w1002 w1011 w1019 w1028 w1037 w1047 w1056 w1065 w1074 w1083 w1092] -> w966
                    tunnel: w965 -> [w974 w983 w992 w1001 w1010 w1020 w1029 w1038 w1046 w1055 w1064 w1073 w1082 w1091]
                    frame 0, Default {
                      n225 = call-poly <vilib>:"Read Key.vi"("section"=w980, "error in (no error)"=w979, "key"=w976, "refnum"=w982) -> ("error out"=w978:errorcluster, "value"=w977:string, "refnum out"=w981:T2)  [unwired: 4 in, 1 out]
                      n226 = Bundle By Name(cluster=w974, "規格"=w977) -> (w975:T1)
                    }
                    frame 1 {
                      n227 = call-poly <vilib>:"Read Key.vi"("section"=w989, "error in (no error)"=w988, "key"=w985, "refnum"=w991) -> ("error out"=w987:errorcluster, "value"=w986:string, "refnum out"=w990:T2)  [unwired: 4 in, 1 out]
                      n228 = Bundle By Name(cluster=w983, "規格上限"=w986) -> (w984:T1)
                    }
                    frame 2 {
                      n229 = call-poly <vilib>:"Read Key.vi"("section"=w998, "error in (no error)"=w997, "key"=w994, "refnum"=w1000) -> ("error out"=w996:errorcluster, "value"=w995:string, "refnum out"=w999:T2)  [unwired: 4 in, 1 out]
                      n230 = Bundle By Name(cluster=w992, "規格下限"=w995) -> (w993:T1)
                    }
                    frame 3 {
                      n231 = call-poly <vilib>:"Read Key.vi"("section"=w1007, "error in (no error)"=w1006, "key"=w1003, "refnum"=w1009) -> ("error out"=w1005:errorcluster, "value"=w1004:i32, "refnum out"=w1008:T2)  [unwired: 4 in, 1 out]
                      n232 = Bundle By Name(cluster=w1001, "ポートNo."=w1004) -> (w1002:T1)
                    }
                    frame 4 {
                      n233 = call-poly <vilib>:"Read Key.vi"("section"=w1016, "error in (no error)"=w1015, "key"=w1012, "refnum"=w1018) -> ("error out"=w1014:errorcluster, "value"=w1013:i32, "refnum out"=w1017:T2)  [unwired: 4 in, 1 out]
                      n234 = Bundle By Name(cluster=w1010, "測定モード"=w1013) -> (w1011:T1)
                    }
                    frame 5 {
                      n235 = call-poly <vilib>:"Read Key.vi"("section"=w1025, "error in (no error)"=w1024, "key"=w1021, "refnum"=w1027) -> ("error out"=w1023:errorcluster, "value"=w1022:string, "refnum out"=w1026:T2)  [unwired: 4 in, 1 out]
                      n236 = Bundle By Name(cluster=w1020, "規格単位"=w1022) -> (w1019:T1)
                    }
                    frame 6 {
                      n237 = call-poly <vilib>:"Read Key.vi"("section"=w1034, "error in (no error)"=w1033, "key"=w1030, "refnum"=w1036) -> ("error out"=w1032:errorcluster, "value"=w1031:string, "refnum out"=w1035:T2)  [unwired: 4 in, 1 out]
                      n238 = Bundle By Name(cluster=w1029, "品質チェック項目"=w1031) -> (w1028:T1)
                    }
                    frame 7 {
                      n239 = call-poly <vilib>:"Read Key.vi"("section"=w1043, "error in (no error)"=w1042, "key"=w1039, "refnum"=w1045) -> ("error out"=w1041:errorcluster, "value"=w1040:i32, "refnum out"=w1044:T2)  [unwired: 4 in, 1 out]
                      n240 = Bundle By Name(cluster=w1038, "測定周期"=w1040) -> (w1037:T1)
                    }
                    frame 8 {
                      n241 = call-poly <vilib>:"Read Key.vi"("section"=w1052, "error in (no error)"=w1051, "key"=w1048, "refnum"=w1054) -> ("error out"=w1050:errorcluster, "value"=w1049:string, "refnum out"=w1053:T2)  [unwired: 4 in, 1 out]
                      n242 = Bundle By Name(cluster=w1046, "実測値MAX"=w1049) -> (w1047:T1)
                    }
                    frame 9 {
                      n243 = call-poly <vilib>:"Read Key.vi"("section"=w1061, "error in (no error)"=w1060, "key"=w1057, "refnum"=w1063) -> ("error out"=w1059:errorcluster, "value"=w1058:string, "refnum out"=w1062:T2)  [unwired: 4 in, 1 out]
                      n244 = Bundle By Name(cluster=w1055, "実測値MIN"=w1058) -> (w1056:T1)
                    }
                    frame 10 {
                      n245 = call-poly <vilib>:"Read Key.vi"("section"=w1070, "error in (no error)"=w1069, "key"=w1066, "refnum"=w1072) -> ("error out"=w1068:errorcluster, "value"=w1067:string, "refnum out"=w1071:T2)  [unwired: 4 in, 1 out]
                      n246 = Bundle By Name(cluster=w1064, "実測値(MAX)"=w1067) -> (w1065:T1)
                    }
                    frame 11 {
                      n247 = call-poly <vilib>:"Read Key.vi"("section"=w1079, "error in (no error)"=w1078, "key"=w1075, "refnum"=w1081) -> ("error out"=w1077:errorcluster, "value"=w1076:string, "refnum out"=w1080:T2)  [unwired: 4 in, 1 out]
                      n248 = Bundle By Name(cluster=w1073, "実測値(MIN)"=w1076) -> (w1074:T1)
                    }
                    frame 12 {
                      n249 = call-poly <vilib>:"Read Key.vi"("section"=w1088, "error in (no error)"=w1087, "key"=w1084, "refnum"=w1090) -> ("error out"=w1086:errorcluster, "value"=w1085:bool, "refnum out"=w1089:T2)  [unwired: 4 in, 1 out]
                      n250 = Bundle By Name(cluster=w1082, "測定画面表示ボタン"=w1085) -> (w1083:T1)
                    }
                    frame 13 {
                      n251 = call-poly <vilib>:"Read Key.vi"("section"=w1097, "error in (no error)"=w1096, "key"=w1093, "refnum"=w1099) -> ("error out"=w1095:errorcluster, "value"=w1094:string, "refnum out"=w1098:T2)  [unwired: 4 in, 1 out]
                      n252 = Bundle By Name(cluster=w1091, "ゲージポートNo"=w1094) -> (w1092:T1)
                    }
                  }
                  n253 = local write "メイン設定_設定 7"(w966) -> ()
                }
              }
              frame #1 {
                n254 = local read "メイン設定_設定 7"() -> (w1100:T1)
              }
            }
            n255 = Replace Array Subset(array=w952, new element=w950, index=6) -> (w951:T1[])
          }
          frame 7 {
            # "③"
            n256 = flat-sequence {
              tunnel: w1112 -> [w1114]
              tunnel: w1111 -> [w1113]
              tunnel: [w1118] -> w1108
              tunnel: [w1117] -> w1107
              tunnel: [w1255] -> w1109
              tunnel: [w1256] -> w1110
              tunnel: w1108 -> [w1256]
              tunnel: w1107 -> [w1255]
              tunnel: [w1254] -> w1104
              frame #0 {
                # "④"
                # "setting.iniファイルからの設定項目の読み取り"
                n257 = for {
                  tunnel: "設定8" -> [w1126]
                  tunnel: string[] ["規格", "規格上限", "規格下限", "ポートNo.", "測定モード", "規格単位", "品質チェック項目", "測定周期", "実測MAX", "実測MIN", "実測(MAX)", "実測(MIN)", "測定画面表示ボタン", "ゲージポートNo.", ""] -> [w1121] mode=indexing
                  tunnel: w1113 -> [w1123]
                  tunnel: [w1122] -> w1117
                  tunnel: w1114 -> [w1127]
                  tunnel: [w1125] -> w1118
                  i -> [w1124]
                  n258 = local read "メイン設定_設定 8"() -> (w1119:T1)
                  n259 = case shown="1" w1124 {
                    tunnel: w1127 -> [w1136 w1145 w1154 w1163 w1172 w1181 w1190 w1199 w1208 w1217 w1226 w1235 w1244 w1253]
                    tunnel: [w1135 w1144 w1153 w1162 w1171 w1180 w1189 w1198 w1207 w1216 w1225 w1234 w1243 w1252] -> w1125
                    tunnel: w1126 -> [w1134 w1143 w1152 w1161 w1170 w1179 w1188 w1197 w1206 w1215 w1224 w1233 w1242 w1251]
                    tunnel: w1123 -> [w1133 w1142 w1151 w1160 w1169 w1178 w1187 w1196 w1205 w1214 w1223 w1232 w1241 w1250]
                    tunnel: [w1132 w1141 w1150 w1159 w1168 w1177 w1186 w1195 w1204 w1213 w1222 w1231 w1240 w1249] -> w1122
                    tunnel: w1121 -> [w1130 w1139 w1148 w1157 w1166 w1175 w1184 w1193 w1202 w1211 w1220 w1229 w1238 w1247]
                    tunnel: [w1129 w1138 w1147 w1156 w1165 w1173 w1182 w1191 w1201 w1210 w1219 w1228 w1237 w1246] -> w1120
                    tunnel: w1119 -> [w1128 w1137 w1146 w1155 w1164 w1174 w1183 w1192 w1200 w1209 w1218 w1227 w1236 w1245]
                    frame 0, Default {
                      n260 = call-poly <vilib>:"Read Key.vi"("section"=w1134, "error in (no error)"=w1133, "key"=w1130, "refnum"=w1136) -> ("error out"=w1132:errorcluster, "value"=w1131:string, "refnum out"=w1135:T2)  [unwired: 4 in, 1 out]
                      n261 = Bundle By Name(cluster=w1128, "規格"=w1131) -> (w1129:T1)
                    }
                    frame 1 {
                      n262 = call-poly <vilib>:"Read Key.vi"("section"=w1143, "error in (no error)"=w1142, "key"=w1139, "refnum"=w1145) -> ("error out"=w1141:errorcluster, "value"=w1140:string, "refnum out"=w1144:T2)  [unwired: 4 in, 1 out]
                      n263 = Bundle By Name(cluster=w1137, "規格上限"=w1140) -> (w1138:T1)
                    }
                    frame 2 {
                      n264 = call-poly <vilib>:"Read Key.vi"("section"=w1152, "error in (no error)"=w1151, "key"=w1148, "refnum"=w1154) -> ("error out"=w1150:errorcluster, "value"=w1149:string, "refnum out"=w1153:T2)  [unwired: 4 in, 1 out]
                      n265 = Bundle By Name(cluster=w1146, "規格下限"=w1149) -> (w1147:T1)
                    }
                    frame 3 {
                      n266 = call-poly <vilib>:"Read Key.vi"("section"=w1161, "error in (no error)"=w1160, "key"=w1157, "refnum"=w1163) -> ("error out"=w1159:errorcluster, "value"=w1158:i32, "refnum out"=w1162:T2)  [unwired: 4 in, 1 out]
                      n267 = Bundle By Name(cluster=w1155, "ポートNo."=w1158) -> (w1156:T1)
                    }
                    frame 4 {
                      n268 = call-poly <vilib>:"Read Key.vi"("section"=w1170, "error in (no error)"=w1169, "key"=w1166, "refnum"=w1172) -> ("error out"=w1168:errorcluster, "value"=w1167:i32, "refnum out"=w1171:T2)  [unwired: 4 in, 1 out]
                      n269 = Bundle By Name(cluster=w1164, "測定モード"=w1167) -> (w1165:T1)
                    }
                    frame 5 {
                      n270 = call-poly <vilib>:"Read Key.vi"("section"=w1179, "error in (no error)"=w1178, "key"=w1175, "refnum"=w1181) -> ("error out"=w1177:errorcluster, "value"=w1176:string, "refnum out"=w1180:T2)  [unwired: 4 in, 1 out]
                      n271 = Bundle By Name(cluster=w1174, "規格単位"=w1176) -> (w1173:T1)
                    }
                    frame 6 {
                      n272 = call-poly <vilib>:"Read Key.vi"("section"=w1188, "error in (no error)"=w1187, "key"=w1184, "refnum"=w1190) -> ("error out"=w1186:errorcluster, "value"=w1185:string, "refnum out"=w1189:T2)  [unwired: 4 in, 1 out]
                      n273 = Bundle By Name(cluster=w1183, "品質チェック項目"=w1185) -> (w1182:T1)
                    }
                    frame 7 {
                      n274 = call-poly <vilib>:"Read Key.vi"("section"=w1197, "error in (no error)"=w1196, "key"=w1193, "refnum"=w1199) -> ("error out"=w1195:errorcluster, "value"=w1194:i32, "refnum out"=w1198:T2)  [unwired: 4 in, 1 out]
                      n275 = Bundle By Name(cluster=w1192, "測定周期"=w1194) -> (w1191:T1)
                    }
                    frame 8 {
                      n276 = call-poly <vilib>:"Read Key.vi"("section"=w1206, "error in (no error)"=w1205, "key"=w1202, "refnum"=w1208) -> ("error out"=w1204:errorcluster, "value"=w1203:string, "refnum out"=w1207:T2)  [unwired: 4 in, 1 out]
                      n277 = Bundle By Name(cluster=w1200, "実測値MAX"=w1203) -> (w1201:T1)
                    }
                    frame 9 {
                      n278 = call-poly <vilib>:"Read Key.vi"("section"=w1215, "error in (no error)"=w1214, "key"=w1211, "refnum"=w1217) -> ("error out"=w1213:errorcluster, "value"=w1212:string, "refnum out"=w1216:T2)  [unwired: 4 in, 1 out]
                      n279 = Bundle By Name(cluster=w1209, "実測値MIN"=w1212) -> (w1210:T1)
                    }
                    frame 10 {
                      n280 = call-poly <vilib>:"Read Key.vi"("section"=w1224, "error in (no error)"=w1223, "key"=w1220, "refnum"=w1226) -> ("error out"=w1222:errorcluster, "value"=w1221:string, "refnum out"=w1225:T2)  [unwired: 4 in, 1 out]
                      n281 = Bundle By Name(cluster=w1218, "実測値(MAX)"=w1221) -> (w1219:T1)
                    }
                    frame 11 {
                      n282 = call-poly <vilib>:"Read Key.vi"("section"=w1233, "error in (no error)"=w1232, "key"=w1229, "refnum"=w1235) -> ("error out"=w1231:errorcluster, "value"=w1230:string, "refnum out"=w1234:T2)  [unwired: 4 in, 1 out]
                      n283 = Bundle By Name(cluster=w1227, "実測値(MIN)"=w1230) -> (w1228:T1)
                    }
                    frame 12 {
                      n284 = call-poly <vilib>:"Read Key.vi"("section"=w1242, "error in (no error)"=w1241, "key"=w1238, "refnum"=w1244) -> ("error out"=w1240:errorcluster, "value"=w1239:bool, "refnum out"=w1243:T2)  [unwired: 4 in, 1 out]
                      n285 = Bundle By Name(cluster=w1236, "測定画面表示ボタン"=w1239) -> (w1237:T1)
                    }
                    frame 13 {
                      n286 = call-poly <vilib>:"Read Key.vi"("section"=w1251, "error in (no error)"=w1250, "key"=w1247, "refnum"=w1253) -> ("error out"=w1249:errorcluster, "value"=w1248:string, "refnum out"=w1252:T2)  [unwired: 4 in, 1 out]
                      n287 = Bundle By Name(cluster=w1245, "ゲージポートNo"=w1248) -> (w1246:T1)
                    }
                  }
                  n288 = local write "メイン設定_設定 8"(w1120) -> ()
                }
              }
              frame #1 {
                n289 = local read "メイン設定_設定 8"() -> (w1254:T1)
              }
            }
            n290 = Replace Array Subset(array=w1106, new element=w1104, index=7) -> (w1105:T1[])
          }
          frame 8 {
            # "③"
            n291 = flat-sequence {
              tunnel: w1266 -> [w1268]
              tunnel: w1265 -> [w1267]
              tunnel: [w1272] -> w1262
              tunnel: [w1271] -> w1261
              tunnel: [w1409] -> w1263
              tunnel: [w1410] -> w1264
              tunnel: w1262 -> [w1410]
              tunnel: w1261 -> [w1409]
              tunnel: [w1408] -> w1258
              frame #0 {
                # "④"
                # "setting.iniファイルからの設定項目の読み取り"
                n292 = for {
                  tunnel: "設定9" -> [w1280]
                  tunnel: string[] ["規格", "規格上限", "規格下限", "ポートNo.", "測定モード", "規格単位", "品質チェック項目", "測定周期", "実測MAX", "実測MIN", "実測(MAX)", "実測(MIN)", "測定画面表示ボタン", "ゲージポートNo.", ""] -> [w1275] mode=indexing
                  tunnel: w1267 -> [w1277]
                  tunnel: [w1276] -> w1271
                  tunnel: w1268 -> [w1281]
                  tunnel: [w1279] -> w1272
                  i -> [w1278]
                  n293 = local read "メイン設定_設定 9"() -> (w1273:T1)
                  n294 = case shown="1" w1278 {
                    tunnel: w1281 -> [w1290 w1299 w1308 w1317 w1326 w1335 w1344 w1353 w1362 w1371 w1380 w1389 w1398 w1407]
                    tunnel: [w1289 w1298 w1307 w1316 w1325 w1334 w1343 w1352 w1361 w1370 w1379 w1388 w1397 w1406] -> w1279
                    tunnel: w1280 -> [w1288 w1297 w1306 w1315 w1324 w1333 w1342 w1351 w1360 w1369 w1378 w1387 w1396 w1405]
                    tunnel: w1277 -> [w1287 w1296 w1305 w1314 w1323 w1332 w1341 w1350 w1359 w1368 w1377 w1386 w1395 w1404]
                    tunnel: [w1286 w1295 w1304 w1313 w1322 w1331 w1340 w1349 w1358 w1367 w1376 w1385 w1394 w1403] -> w1276
                    tunnel: w1275 -> [w1284 w1293 w1302 w1311 w1320 w1329 w1338 w1347 w1356 w1365 w1374 w1383 w1392 w1401]
                    tunnel: [w1283 w1292 w1301 w1310 w1319 w1327 w1336 w1345 w1355 w1364 w1373 w1382 w1391 w1400] -> w1274
                    tunnel: w1273 -> [w1282 w1291 w1300 w1309 w1318 w1328 w1337 w1346 w1354 w1363 w1372 w1381 w1390 w1399]
                    frame 0, Default {
                      n295 = call-poly <vilib>:"Read Key.vi"("section"=w1288, "error in (no error)"=w1287, "key"=w1284, "refnum"=w1290) -> ("error out"=w1286:errorcluster, "value"=w1285:string, "refnum out"=w1289:T2)  [unwired: 4 in, 1 out]
                      n296 = Bundle By Name(cluster=w1282, "規格"=w1285) -> (w1283:T1)
                    }
                    frame 1 {
                      n297 = call-poly <vilib>:"Read Key.vi"("section"=w1297, "error in (no error)"=w1296, "key"=w1293, "refnum"=w1299) -> ("error out"=w1295:errorcluster, "value"=w1294:string, "refnum out"=w1298:T2)  [unwired: 4 in, 1 out]
                      n298 = Bundle By Name(cluster=w1291, "規格上限"=w1294) -> (w1292:T1)
                    }
                    frame 2 {
                      n299 = call-poly <vilib>:"Read Key.vi"("section"=w1306, "error in (no error)"=w1305, "key"=w1302, "refnum"=w1308) -> ("error out"=w1304:errorcluster, "value"=w1303:string, "refnum out"=w1307:T2)  [unwired: 4 in, 1 out]
                      n300 = Bundle By Name(cluster=w1300, "規格下限"=w1303) -> (w1301:T1)
                    }
                    frame 3 {
                      n301 = call-poly <vilib>:"Read Key.vi"("section"=w1315, "error in (no error)"=w1314, "key"=w1311, "refnum"=w1317) -> ("error out"=w1313:errorcluster, "value"=w1312:i32, "refnum out"=w1316:T2)  [unwired: 4 in, 1 out]
                      n302 = Bundle By Name(cluster=w1309, "ポートNo."=w1312) -> (w1310:T1)
                    }
                    frame 4 {
                      n303 = call-poly <vilib>:"Read Key.vi"("section"=w1324, "error in (no error)"=w1323, "key"=w1320, "refnum"=w1326) -> ("error out"=w1322:errorcluster, "value"=w1321:i32, "refnum out"=w1325:T2)  [unwired: 4 in, 1 out]
                      n304 = Bundle By Name(cluster=w1318, "測定モード"=w1321) -> (w1319:T1)
                    }
                    frame 5 {
                      n305 = call-poly <vilib>:"Read Key.vi"("section"=w1333, "error in (no error)"=w1332, "key"=w1329, "refnum"=w1335) -> ("error out"=w1331:errorcluster, "value"=w1330:string, "refnum out"=w1334:T2)  [unwired: 4 in, 1 out]
                      n306 = Bundle By Name(cluster=w1328, "規格単位"=w1330) -> (w1327:T1)
                    }
                    frame 6 {
                      n307 = call-poly <vilib>:"Read Key.vi"("section"=w1342, "error in (no error)"=w1341, "key"=w1338, "refnum"=w1344) -> ("error out"=w1340:errorcluster, "value"=w1339:string, "refnum out"=w1343:T2)  [unwired: 4 in, 1 out]
                      n308 = Bundle By Name(cluster=w1337, "品質チェック項目"=w1339) -> (w1336:T1)
                    }
                    frame 7 {
                      n309 = call-poly <vilib>:"Read Key.vi"("section"=w1351, "error in (no error)"=w1350, "key"=w1347, "refnum"=w1353) -> ("error out"=w1349:errorcluster, "value"=w1348:i32, "refnum out"=w1352:T2)  [unwired: 4 in, 1 out]
                      n310 = Bundle By Name(cluster=w1346, "測定周期"=w1348) -> (w1345:T1)
                    }
                    frame 8 {
                      n311 = call-poly <vilib>:"Read Key.vi"("section"=w1360, "error in (no error)"=w1359, "key"=w1356, "refnum"=w1362) -> ("error out"=w1358:errorcluster, "value"=w1357:string, "refnum out"=w1361:T2)  [unwired: 4 in, 1 out]
                      n312 = Bundle By Name(cluster=w1354, "実測値MAX"=w1357) -> (w1355:T1)
                    }
                    frame 9 {
                      n313 = call-poly <vilib>:"Read Key.vi"("section"=w1369, "error in (no error)"=w1368, "key"=w1365, "refnum"=w1371) -> ("error out"=w1367:errorcluster, "value"=w1366:string, "refnum out"=w1370:T2)  [unwired: 4 in, 1 out]
                      n314 = Bundle By Name(cluster=w1363, "実測値MIN"=w1366) -> (w1364:T1)
                    }
                    frame 10 {
                      n315 = call-poly <vilib>:"Read Key.vi"("section"=w1378, "error in (no error)"=w1377, "key"=w1374, "refnum"=w1380) -> ("error out"=w1376:errorcluster, "value"=w1375:string, "refnum out"=w1379:T2)  [unwired: 4 in, 1 out]
                      n316 = Bundle By Name(cluster=w1372, "実測値(MAX)"=w1375) -> (w1373:T1)
                    }
                    frame 11 {
                      n317 = call-poly <vilib>:"Read Key.vi"("section"=w1387, "error in (no error)"=w1386, "key"=w1383, "refnum"=w1389) -> ("error out"=w1385:errorcluster, "value"=w1384:string, "refnum out"=w1388:T2)  [unwired: 4 in, 1 out]
                      n318 = Bundle By Name(cluster=w1381, "実測値(MIN)"=w1384) -> (w1382:T1)
                    }
                    frame 12 {
                      n319 = call-poly <vilib>:"Read Key.vi"("section"=w1396, "error in (no error)"=w1395, "key"=w1392, "refnum"=w1398) -> ("error out"=w1394:errorcluster, "value"=w1393:bool, "refnum out"=w1397:T2)  [unwired: 4 in, 1 out]
                      n320 = Bundle By Name(cluster=w1390, "測定画面表示ボタン"=w1393) -> (w1391:T1)
                    }
                    frame 13 {
                      n321 = call-poly <vilib>:"Read Key.vi"("section"=w1405, "error in (no error)"=w1404, "key"=w1401, "refnum"=w1407) -> ("error out"=w1403:errorcluster, "value"=w1402:string, "refnum out"=w1406:T2)  [unwired: 4 in, 1 out]
                      n322 = Bundle By Name(cluster=w1399, "ゲージポートNo"=w1402) -> (w1400:T1)
                    }
                  }
                  n323 = local write "メイン設定_設定 9"(w1274) -> ()
                }
              }
              frame #1 {
                n324 = local read "メイン設定_設定 9"() -> (w1408:T1)
              }
            }
            n325 = Replace Array Subset(array=w1260, new element=w1258, index=8) -> (w1259:T1[])
          }
          frame 9 {
            # "③"
            n326 = flat-sequence {
              tunnel: w1420 -> [w1422]
              tunnel: w1419 -> [w1421]
              tunnel: [w1426] -> w1416
              tunnel: [w1425] -> w1415
              tunnel: [w1563] -> w1417
              tunnel: [w1564] -> w1418
              tunnel: w1416 -> [w1564]
              tunnel: w1415 -> [w1563]
              tunnel: [w1562] -> w1412
              frame #0 {
                # "④"
                # "setting.iniファイルからの設定項目の読み取り"
                n327 = for {
                  tunnel: "設定10" -> [w1434]
                  tunnel: string[] ["規格", "規格上限", "規格下限", "ポートNo.", "測定モード", "規格単位", "品質チェック項目", "測定周期", "実測MAX", "実測MIN", "実測(MAX)", "実測(MIN)", "測定画面表示ボタン", "ゲージポートNo.", ""] -> [w1429] mode=indexing
                  tunnel: w1421 -> [w1431]
                  tunnel: [w1430] -> w1425
                  tunnel: w1422 -> [w1435]
                  tunnel: [w1433] -> w1426
                  i -> [w1432]
                  n328 = local read "メイン設定_設定 10"() -> (w1427:T1)
                  n329 = case shown="1" w1432 {
                    tunnel: w1435 -> [w1444 w1453 w1462 w1471 w1480 w1489 w1498 w1507 w1516 w1525 w1534 w1543 w1552 w1561]
                    tunnel: [w1443 w1452 w1461 w1470 w1479 w1488 w1497 w1506 w1515 w1524 w1533 w1542 w1551 w1560] -> w1433
                    tunnel: w1434 -> [w1442 w1451 w1460 w1469 w1478 w1487 w1496 w1505 w1514 w1523 w1532 w1541 w1550 w1559]
                    tunnel: w1431 -> [w1441 w1450 w1459 w1468 w1477 w1486 w1495 w1504 w1513 w1522 w1531 w1540 w1549 w1558]
                    tunnel: [w1440 w1449 w1458 w1467 w1476 w1485 w1494 w1503 w1512 w1521 w1530 w1539 w1548 w1557] -> w1430
                    tunnel: w1429 -> [w1438 w1447 w1456 w1465 w1474 w1483 w1492 w1501 w1510 w1519 w1528 w1537 w1546 w1555]
                    tunnel: [w1437 w1446 w1455 w1464 w1473 w1481 w1490 w1499 w1509 w1518 w1527 w1536 w1545 w1554] -> w1428
                    tunnel: w1427 -> [w1436 w1445 w1454 w1463 w1472 w1482 w1491 w1500 w1508 w1517 w1526 w1535 w1544 w1553]
                    frame 0, Default {
                      n330 = call-poly <vilib>:"Read Key.vi"("section"=w1442, "error in (no error)"=w1441, "key"=w1438, "refnum"=w1444) -> ("error out"=w1440:errorcluster, "value"=w1439:string, "refnum out"=w1443:T2)  [unwired: 4 in, 1 out]
                      n331 = Bundle By Name(cluster=w1436, "規格"=w1439) -> (w1437:T1)
                    }
                    frame 1 {
                      n332 = call-poly <vilib>:"Read Key.vi"("section"=w1451, "error in (no error)"=w1450, "key"=w1447, "refnum"=w1453) -> ("error out"=w1449:errorcluster, "value"=w1448:string, "refnum out"=w1452:T2)  [unwired: 4 in, 1 out]
                      n333 = Bundle By Name(cluster=w1445, "規格上限"=w1448) -> (w1446:T1)
                    }
                    frame 2 {
                      n334 = call-poly <vilib>:"Read Key.vi"("section"=w1460, "error in (no error)"=w1459, "key"=w1456, "refnum"=w1462) -> ("error out"=w1458:errorcluster, "value"=w1457:string, "refnum out"=w1461:T2)  [unwired: 4 in, 1 out]
                      n335 = Bundle By Name(cluster=w1454, "規格下限"=w1457) -> (w1455:T1)
                    }
                    frame 3 {
                      n336 = call-poly <vilib>:"Read Key.vi"("section"=w1469, "error in (no error)"=w1468, "key"=w1465, "refnum"=w1471) -> ("error out"=w1467:errorcluster, "value"=w1466:i32, "refnum out"=w1470:T2)  [unwired: 4 in, 1 out]
                      n337 = Bundle By Name(cluster=w1463, "ポートNo."=w1466) -> (w1464:T1)
                    }
                    frame 4 {
                      n338 = call-poly <vilib>:"Read Key.vi"("section"=w1478, "error in (no error)"=w1477, "key"=w1474, "refnum"=w1480) -> ("error out"=w1476:errorcluster, "value"=w1475:i32, "refnum out"=w1479:T2)  [unwired: 4 in, 1 out]
                      n339 = Bundle By Name(cluster=w1472, "測定モード"=w1475) -> (w1473:T1)
                    }
                    frame 5 {
                      n340 = call-poly <vilib>:"Read Key.vi"("section"=w1487, "error in (no error)"=w1486, "key"=w1483, "refnum"=w1489) -> ("error out"=w1485:errorcluster, "value"=w1484:string, "refnum out"=w1488:T2)  [unwired: 4 in, 1 out]
                      n341 = Bundle By Name(cluster=w1482, "規格単位"=w1484) -> (w1481:T1)
                    }
                    frame 6 {
                      n342 = call-poly <vilib>:"Read Key.vi"("section"=w1496, "error in (no error)"=w1495, "key"=w1492, "refnum"=w1498) -> ("error out"=w1494:errorcluster, "value"=w1493:string, "refnum out"=w1497:T2)  [unwired: 4 in, 1 out]
                      n343 = Bundle By Name(cluster=w1491, "品質チェック項目"=w1493) -> (w1490:T1)
                    }
                    frame 7 {
                      n344 = call-poly <vilib>:"Read Key.vi"("section"=w1505, "error in (no error)"=w1504, "key"=w1501, "refnum"=w1507) -> ("error out"=w1503:errorcluster, "value"=w1502:i32, "refnum out"=w1506:T2)  [unwired: 4 in, 1 out]
                      n345 = Bundle By Name(cluster=w1500, "測定周期"=w1502) -> (w1499:T1)
                    }
                    frame 8 {
                      n346 = call-poly <vilib>:"Read Key.vi"("section"=w1514, "error in (no error)"=w1513, "key"=w1510, "refnum"=w1516) -> ("error out"=w1512:errorcluster, "value"=w1511:string, "refnum out"=w1515:T2)  [unwired: 4 in, 1 out]
                      n347 = Bundle By Name(cluster=w1508, "実測値MAX"=w1511) -> (w1509:T1)
                    }
                    frame 9 {
                      n348 = call-poly <vilib>:"Read Key.vi"("section"=w1523, "error in (no error)"=w1522, "key"=w1519, "refnum"=w1525) -> ("error out"=w1521:errorcluster, "value"=w1520:string, "refnum out"=w1524:T2)  [unwired: 4 in, 1 out]
                      n349 = Bundle By Name(cluster=w1517, "実測値MIN"=w1520) -> (w1518:T1)
                    }
                    frame 10 {
                      n350 = call-poly <vilib>:"Read Key.vi"("section"=w1532, "error in (no error)"=w1531, "key"=w1528, "refnum"=w1534) -> ("error out"=w1530:errorcluster, "value"=w1529:string, "refnum out"=w1533:T2)  [unwired: 4 in, 1 out]
                      n351 = Bundle By Name(cluster=w1526, "実測値(MAX)"=w1529) -> (w1527:T1)
                    }
                    frame 11 {
                      n352 = call-poly <vilib>:"Read Key.vi"("section"=w1541, "error in (no error)"=w1540, "key"=w1537, "refnum"=w1543) -> ("error out"=w1539:errorcluster, "value"=w1538:string, "refnum out"=w1542:T2)  [unwired: 4 in, 1 out]
                      n353 = Bundle By Name(cluster=w1535, "実測値(MIN)"=w1538) -> (w1536:T1)
                    }
                    frame 12 {
                      n354 = call-poly <vilib>:"Read Key.vi"("section"=w1550, "error in (no error)"=w1549, "key"=w1546, "refnum"=w1552) -> ("error out"=w1548:errorcluster, "value"=w1547:bool, "refnum out"=w1551:T2)  [unwired: 4 in, 1 out]
                      n355 = Bundle By Name(cluster=w1544, "測定画面表示ボタン"=w1547) -> (w1545:T1)
                    }
                    frame 13 {
                      n356 = call-poly <vilib>:"Read Key.vi"("section"=w1559, "error in (no error)"=w1558, "key"=w1555, "refnum"=w1561) -> ("error out"=w1557:errorcluster, "value"=w1556:string, "refnum out"=w1560:T2)  [unwired: 4 in, 1 out]
                      n357 = Bundle By Name(cluster=w1553, "ゲージポートNo"=w1556) -> (w1554:T1)
                    }
                  }
                  n358 = local write "メイン設定_設定 10"(w1428) -> ()
                }
              }
              frame #1 {
                n359 = local read "メイン設定_設定 10"() -> (w1562:T1)
              }
            }
            n360 = Replace Array Subset(array=w1414, new element=w1412, index=9) -> (w1413:T1[])
          }
          frame 10 {
            # "③"
            n361 = flat-sequence {
              tunnel: w1574 -> [w1576]
              tunnel: w1573 -> [w1575]
              tunnel: [w1580] -> w1570
              tunnel: [w1579] -> w1569
              tunnel: [w1717] -> w1571
              tunnel: [w1718] -> w1572
              tunnel: w1570 -> [w1718]
              tunnel: w1569 -> [w1717]
              tunnel: [w1716] -> w1566
              frame #0 {
                # "④"
                # "setting.iniファイルからの設定項目の読み取り"
                n362 = for {
                  tunnel: "設定11" -> [w1588]
                  tunnel: string[] ["規格", "規格上限", "規格下限", "ポートNo.", "測定モード", "規格単位", "品質チェック項目", "測定周期", "実測MAX", "実測MIN", "実測(MAX)", "実測(MIN)", "測定画面表示ボタン", "ゲージポートNo.", ""] -> [w1583] mode=indexing
                  tunnel: w1575 -> [w1585]
                  tunnel: [w1584] -> w1579
                  tunnel: w1576 -> [w1589]
                  tunnel: [w1587] -> w1580
                  i -> [w1586]
                  n363 = local read "メイン設定_設定 11"() -> (w1581:T1)
                  n364 = case shown="1" w1586 {
                    tunnel: w1589 -> [w1598 w1607 w1616 w1625 w1634 w1643 w1652 w1661 w1670 w1679 w1688 w1697 w1706 w1715]
                    tunnel: [w1597 w1606 w1615 w1624 w1633 w1642 w1651 w1660 w1669 w1678 w1687 w1696 w1705 w1714] -> w1587
                    tunnel: w1588 -> [w1596 w1605 w1614 w1623 w1632 w1641 w1650 w1659 w1668 w1677 w1686 w1695 w1704 w1713]
                    tunnel: w1585 -> [w1595 w1604 w1613 w1622 w1631 w1640 w1649 w1658 w1667 w1676 w1685 w1694 w1703 w1712]
                    tunnel: [w1594 w1603 w1612 w1621 w1630 w1639 w1648 w1657 w1666 w1675 w1684 w1693 w1702 w1711] -> w1584
                    tunnel: w1583 -> [w1592 w1601 w1610 w1619 w1628 w1637 w1646 w1655 w1664 w1673 w1682 w1691 w1700 w1709]
                    tunnel: [w1591 w1600 w1609 w1618 w1627 w1635 w1644 w1653 w1663 w1672 w1681 w1690 w1699 w1708] -> w1582
                    tunnel: w1581 -> [w1590 w1599 w1608 w1617 w1626 w1636 w1645 w1654 w1662 w1671 w1680 w1689 w1698 w1707]
                    frame 0, Default {
                      n365 = call-poly <vilib>:"Read Key.vi"("section"=w1596, "error in (no error)"=w1595, "key"=w1592, "refnum"=w1598) -> ("error out"=w1594:errorcluster, "value"=w1593:string, "refnum out"=w1597:T2)  [unwired: 4 in, 1 out]
                      n366 = Bundle By Name(cluster=w1590, "規格"=w1593) -> (w1591:T1)
                    }
                    frame 1 {
                      n367 = call-poly <vilib>:"Read Key.vi"("section"=w1605, "error in (no error)"=w1604, "key"=w1601, "refnum"=w1607) -> ("error out"=w1603:errorcluster, "value"=w1602:string, "refnum out"=w1606:T2)  [unwired: 4 in, 1 out]
                      n368 = Bundle By Name(cluster=w1599, "規格上限"=w1602) -> (w1600:T1)
                    }
                    frame 2 {
                      n369 = call-poly <vilib>:"Read Key.vi"("section"=w1614, "error in (no error)"=w1613, "key"=w1610, "refnum"=w1616) -> ("error out"=w1612:errorcluster, "value"=w1611:string, "refnum out"=w1615:T2)  [unwired: 4 in, 1 out]
                      n370 = Bundle By Name(cluster=w1608, "規格下限"=w1611) -> (w1609:T1)
                    }
                    frame 3 {
                      n371 = call-poly <vilib>:"Read Key.vi"("section"=w1623, "error in (no error)"=w1622, "key"=w1619, "refnum"=w1625) -> ("error out"=w1621:errorcluster, "value"=w1620:i32, "refnum out"=w1624:T2)  [unwired: 4 in, 1 out]
                      n372 = Bundle By Name(cluster=w1617, "ポートNo."=w1620) -> (w1618:T1)
                    }
                    frame 4 {
                      n373 = call-poly <vilib>:"Read Key.vi"("section"=w1632, "error in (no error)"=w1631, "key"=w1628, "refnum"=w1634) -> ("error out"=w1630:errorcluster, "value"=w1629:i32, "refnum out"=w1633:T2)  [unwired: 4 in, 1 out]
                      n374 = Bundle By Name(cluster=w1626, "測定モード"=w1629) -> (w1627:T1)
                    }
                    frame 5 {
                      n375 = call-poly <vilib>:"Read Key.vi"("section"=w1641, "error in (no error)"=w1640, "key"=w1637, "refnum"=w1643) -> ("error out"=w1639:errorcluster, "value"=w1638:string, "refnum out"=w1642:T2)  [unwired: 4 in, 1 out]
                      n376 = Bundle By Name(cluster=w1636, "規格単位"=w1638) -> (w1635:T1)
                    }
                    frame 6 {
                      n377 = call-poly <vilib>:"Read Key.vi"("section"=w1650, "error in (no error)"=w1649, "key"=w1646, "refnum"=w1652) -> ("error out"=w1648:errorcluster, "value"=w1647:string, "refnum out"=w1651:T2)  [unwired: 4 in, 1 out]
                      n378 = Bundle By Name(cluster=w1645, "品質チェック項目"=w1647) -> (w1644:T1)
                    }
                    frame 7 {
                      n379 = call-poly <vilib>:"Read Key.vi"("section"=w1659, "error in (no error)"=w1658, "key"=w1655, "refnum"=w1661) -> ("error out"=w1657:errorcluster, "value"=w1656:i32, "refnum out"=w1660:T2)  [unwired: 4 in, 1 out]
                      n380 = Bundle By Name(cluster=w1654, "測定周期"=w1656) -> (w1653:T1)
                    }
                    frame 8 {
                      n381 = call-poly <vilib>:"Read Key.vi"("section"=w1668, "error in (no error)"=w1667, "key"=w1664, "refnum"=w1670) -> ("error out"=w1666:errorcluster, "value"=w1665:string, "refnum out"=w1669:T2)  [unwired: 4 in, 1 out]
                      n382 = Bundle By Name(cluster=w1662, "実測値MAX"=w1665) -> (w1663:T1)
                    }
                    frame 9 {
                      n383 = call-poly <vilib>:"Read Key.vi"("section"=w1677, "error in (no error)"=w1676, "key"=w1673, "refnum"=w1679) -> ("error out"=w1675:errorcluster, "value"=w1674:string, "refnum out"=w1678:T2)  [unwired: 4 in, 1 out]
                      n384 = Bundle By Name(cluster=w1671, "実測値MIN"=w1674) -> (w1672:T1)
                    }
                    frame 10 {
                      n385 = call-poly <vilib>:"Read Key.vi"("section"=w1686, "error in (no error)"=w1685, "key"=w1682, "refnum"=w1688) -> ("error out"=w1684:errorcluster, "value"=w1683:string, "refnum out"=w1687:T2)  [unwired: 4 in, 1 out]
                      n386 = Bundle By Name(cluster=w1680, "実測値(MAX)"=w1683) -> (w1681:T1)
                    }
                    frame 11 {
                      n387 = call-poly <vilib>:"Read Key.vi"("section"=w1695, "error in (no error)"=w1694, "key"=w1691, "refnum"=w1697) -> ("error out"=w1693:errorcluster, "value"=w1692:string, "refnum out"=w1696:T2)  [unwired: 4 in, 1 out]
                      n388 = Bundle By Name(cluster=w1689, "実測値(MIN)"=w1692) -> (w1690:T1)
                    }
                    frame 12 {
                      n389 = call-poly <vilib>:"Read Key.vi"("section"=w1704, "error in (no error)"=w1703, "key"=w1700, "refnum"=w1706) -> ("error out"=w1702:errorcluster, "value"=w1701:bool, "refnum out"=w1705:T2)  [unwired: 4 in, 1 out]
                      n390 = Bundle By Name(cluster=w1698, "測定画面表示ボタン"=w1701) -> (w1699:T1)
                    }
                    frame 13 {
                      n391 = call-poly <vilib>:"Read Key.vi"("section"=w1713, "error in (no error)"=w1712, "key"=w1709, "refnum"=w1715) -> ("error out"=w1711:errorcluster, "value"=w1710:string, "refnum out"=w1714:T2)  [unwired: 4 in, 1 out]
                      n392 = Bundle By Name(cluster=w1707, "ゲージポートNo"=w1710) -> (w1708:T1)
                    }
                  }
                  n393 = local write "メイン設定_設定 11"(w1582) -> ()
                }
              }
              frame #1 {
                n394 = local read "メイン設定_設定 11"() -> (w1716:T1)
              }
            }
            n395 = Replace Array Subset(array=w1568, new element=w1566, index=10) -> (w1567:T1[])
          }
          frame 11 {
            # "③"
            n396 = flat-sequence {
              tunnel: w1728 -> [w1730]
              tunnel: w1727 -> [w1729]
              tunnel: [w1734] -> w1724
              tunnel: [w1733] -> w1723
              tunnel: [w1871] -> w1725
              tunnel: [w1872] -> w1726
              tunnel: w1724 -> [w1872]
              tunnel: w1723 -> [w1871]
              tunnel: [w1870] -> w1720
              frame #0 {
                # "④"
                # "setting.iniファイルからの設定項目の読み取り"
                n397 = for {
                  tunnel: "設定12" -> [w1742]
                  tunnel: string[] ["規格", "規格上限", "規格下限", "ポートNo.", "測定モード", "規格単位", "品質チェック項目", "測定周期", "実測MAX", "実測MIN", "実測(MAX)", "実測(MIN)", "測定画面表示ボタン", "ゲージポートNo.", ""] -> [w1737] mode=indexing
                  tunnel: w1729 -> [w1739]
                  tunnel: [w1738] -> w1733
                  tunnel: w1730 -> [w1743]
                  tunnel: [w1741] -> w1734
                  i -> [w1740]
                  n398 = local read "メイン設定_設定 12"() -> (w1735:T1)
                  n399 = case shown="1" w1740 {
                    tunnel: w1743 -> [w1752 w1761 w1770 w1779 w1788 w1797 w1806 w1815 w1824 w1833 w1842 w1851 w1860 w1869]
                    tunnel: [w1751 w1760 w1769 w1778 w1787 w1796 w1805 w1814 w1823 w1832 w1841 w1850 w1859 w1868] -> w1741
                    tunnel: w1742 -> [w1750 w1759 w1768 w1777 w1786 w1795 w1804 w1813 w1822 w1831 w1840 w1849 w1858 w1867]
                    tunnel: w1739 -> [w1749 w1758 w1767 w1776 w1785 w1794 w1803 w1812 w1821 w1830 w1839 w1848 w1857 w1866]
                    tunnel: [w1748 w1757 w1766 w1775 w1784 w1793 w1802 w1811 w1820 w1829 w1838 w1847 w1856 w1865] -> w1738
                    tunnel: w1737 -> [w1746 w1755 w1764 w1773 w1782 w1791 w1800 w1809 w1818 w1827 w1836 w1845 w1854 w1863]
                    tunnel: [w1745 w1754 w1763 w1772 w1781 w1789 w1798 w1807 w1817 w1826 w1835 w1844 w1853 w1862] -> w1736
                    tunnel: w1735 -> [w1744 w1753 w1762 w1771 w1780 w1790 w1799 w1808 w1816 w1825 w1834 w1843 w1852 w1861]
                    frame 0, Default {
                      n400 = call-poly <vilib>:"Read Key.vi"("section"=w1750, "error in (no error)"=w1749, "key"=w1746, "refnum"=w1752) -> ("error out"=w1748:errorcluster, "value"=w1747:string, "refnum out"=w1751:T2)  [unwired: 4 in, 1 out]
                      n401 = Bundle By Name(cluster=w1744, "規格"=w1747) -> (w1745:T1)
                    }
                    frame 1 {
                      n402 = call-poly <vilib>:"Read Key.vi"("section"=w1759, "error in (no error)"=w1758, "key"=w1755, "refnum"=w1761) -> ("error out"=w1757:errorcluster, "value"=w1756:string, "refnum out"=w1760:T2)  [unwired: 4 in, 1 out]
                      n403 = Bundle By Name(cluster=w1753, "規格上限"=w1756) -> (w1754:T1)
                    }
                    frame 2 {
                      n404 = call-poly <vilib>:"Read Key.vi"("section"=w1768, "error in (no error)"=w1767, "key"=w1764, "refnum"=w1770) -> ("error out"=w1766:errorcluster, "value"=w1765:string, "refnum out"=w1769:T2)  [unwired: 4 in, 1 out]
                      n405 = Bundle By Name(cluster=w1762, "規格下限"=w1765) -> (w1763:T1)
                    }
                    frame 3 {
                      n406 = call-poly <vilib>:"Read Key.vi"("section"=w1777, "error in (no error)"=w1776, "key"=w1773, "refnum"=w1779) -> ("error out"=w1775:errorcluster, "value"=w1774:i32, "refnum out"=w1778:T2)  [unwired: 4 in, 1 out]
                      n407 = Bundle By Name(cluster=w1771, "ポートNo."=w1774) -> (w1772:T1)
                    }
                    frame 4 {
                      n408 = call-poly <vilib>:"Read Key.vi"("section"=w1786, "error in (no error)"=w1785, "key"=w1782, "refnum"=w1788) -> ("error out"=w1784:errorcluster, "value"=w1783:i32, "refnum out"=w1787:T2)  [unwired: 4 in, 1 out]
                      n409 = Bundle By Name(cluster=w1780, "測定モード"=w1783) -> (w1781:T1)
                    }
                    frame 5 {
                      n410 = call-poly <vilib>:"Read Key.vi"("section"=w1795, "error in (no error)"=w1794, "key"=w1791, "refnum"=w1797) -> ("error out"=w1793:errorcluster, "value"=w1792:string, "refnum out"=w1796:T2)  [unwired: 4 in, 1 out]
                      n411 = Bundle By Name(cluster=w1790, "規格単位"=w1792) -> (w1789:T1)
                    }
                    frame 6 {
                      n412 = call-poly <vilib>:"Read Key.vi"("section"=w1804, "error in (no error)"=w1803, "key"=w1800, "refnum"=w1806) -> ("error out"=w1802:errorcluster, "value"=w1801:string, "refnum out"=w1805:T2)  [unwired: 4 in, 1 out]
                      n413 = Bundle By Name(cluster=w1799, "品質チェック項目"=w1801) -> (w1798:T1)
                    }
                    frame 7 {
                      n414 = call-poly <vilib>:"Read Key.vi"("section"=w1813, "error in (no error)"=w1812, "key"=w1809, "refnum"=w1815) -> ("error out"=w1811:errorcluster, "value"=w1810:i32, "refnum out"=w1814:T2)  [unwired: 4 in, 1 out]
                      n415 = Bundle By Name(cluster=w1808, "測定周期"=w1810) -> (w1807:T1)
                    }
                    frame 8 {
                      n416 = call-poly <vilib>:"Read Key.vi"("section"=w1822, "error in (no error)"=w1821, "key"=w1818, "refnum"=w1824) -> ("error out"=w1820:errorcluster, "value"=w1819:string, "refnum out"=w1823:T2)  [unwired: 4 in, 1 out]
                      n417 = Bundle By Name(cluster=w1816, "実測値MAX"=w1819) -> (w1817:T1)
                    }
                    frame 9 {
                      n418 = call-poly <vilib>:"Read Key.vi"("section"=w1831, "error in (no error)"=w1830, "key"=w1827, "refnum"=w1833) -> ("error out"=w1829:errorcluster, "value"=w1828:string, "refnum out"=w1832:T2)  [unwired: 4 in, 1 out]
                      n419 = Bundle By Name(cluster=w1825, "実測値MIN"=w1828) -> (w1826:T1)
                    }
                    frame 10 {
                      n420 = call-poly <vilib>:"Read Key.vi"("section"=w1840, "error in (no error)"=w1839, "key"=w1836, "refnum"=w1842) -> ("error out"=w1838:errorcluster, "value"=w1837:string, "refnum out"=w1841:T2)  [unwired: 4 in, 1 out]
                      n421 = Bundle By Name(cluster=w1834, "実測値(MAX)"=w1837) -> (w1835:T1)
                    }
                    frame 11 {
                      n422 = call-poly <vilib>:"Read Key.vi"("section"=w1849, "error in (no error)"=w1848, "key"=w1845, "refnum"=w1851) -> ("error out"=w1847:errorcluster, "value"=w1846:string, "refnum out"=w1850:T2)  [unwired: 4 in, 1 out]
                      n423 = Bundle By Name(cluster=w1843, "実測値(MIN)"=w1846) -> (w1844:T1)
                    }
                    frame 12 {
                      n424 = call-poly <vilib>:"Read Key.vi"("section"=w1858, "error in (no error)"=w1857, "key"=w1854, "refnum"=w1860) -> ("error out"=w1856:errorcluster, "value"=w1855:bool, "refnum out"=w1859:T2)  [unwired: 4 in, 1 out]
                      n425 = Bundle By Name(cluster=w1852, "測定画面表示ボタン"=w1855) -> (w1853:T1)
                    }
                    frame 13 {
                      n426 = call-poly <vilib>:"Read Key.vi"("section"=w1867, "error in (no error)"=w1866, "key"=w1863, "refnum"=w1869) -> ("error out"=w1865:errorcluster, "value"=w1864:string, "refnum out"=w1868:T2)  [unwired: 4 in, 1 out]
                      n427 = Bundle By Name(cluster=w1861, "ゲージポートNo"=w1864) -> (w1862:T1)
                    }
                  }
                  n428 = local write "メイン設定_設定 12"(w1736) -> ()
                }
              }
              frame #1 {
                n429 = local read "メイン設定_設定 12"() -> (w1870:T1)
              }
            }
            n430 = Replace Array Subset(array=w1722, new element=w1720, index=11) -> (w1721:T1[])
          }
          frame 12 {
          }
        }
        "実測設定項目配列_\nメインからの転記" <- w7
        n431 = call <vilib>:"Close Config Data.vi"("error in (no error)"=w10, "refnum"=w11) -> ("error out"=→"setup.iniエラーout":errorcluster)  [unwired: 1 in, 8 out]
      }
    }
    frame #1 {
      # "メインviから設定項目を転記"
      n432 = for {
        N: 32 -> [_]
        i -> [w1880]
        n433 = global read "測定データ転記.vi" "測定転記一時データ"() -> (w1882:string[])
        n434 = Insert Into Array(array=w1882, index=w1880, new element=string[] [""] ("測定転記一時データ")) -> (w1883:string[])
        n435 = global write "測定データ転記.vi" "測定転記一時データ"(w1883) -> ()
      }
      n436 = Wait (ms)(milliseconds to wait=1) -> ()  [unwired: 1 out]
    }
    frame #2 {
      w1884 = 11
      w1901 = 10
      w1902 = 9
      w1919 = 8
      w1920 = 7
      w1937 = 6
      w1938 = 5
      w1955 = 4
      w1956 = 3
      w1965 = 2
      w1973 = 1
      w1981 = 0
      # "メインviから転記された配列のゲージポートNoが空だったらTrue、選択をされていたらFalseを返し処理"
      # "トンネルモード\n最後の値"
      n437 = property on="実測設定項目配列_\nメインからの転記" class="Arr (指定)"() -> ("Value"=w1934:T1[])  [unwired: 2 in, 2 out]
      n438 = property on="実測設定項目配列_\nメインからの転記" class="Arr (指定)"() -> ("Value"=w1923:T1[])  [unwired: 2 in, 2 out]
      n439 = property on="実測設定項目配列_\nメインからの転記" class="Arr (指定)"() -> ("Value"=w1916:T1[])  [unwired: 2 in, 2 out]
      n440 = property on="実測設定項目配列_\nメインからの転記" class="Arr (指定)"() -> ("Value"=w1887:T1[])  [unwired: 2 in, 2 out]
      n441 = property on="実測設定項目配列_\nメインからの転記" class="Arr (指定)"() -> ("Value"=w1959:T1[])  [unwired: 2 in, 2 out]
      n442 = property on="実測設定項目配列_\nメインからの転記" class="Arr (指定)"() -> ("Value"=w1952:T1[])  [unwired: 2 in, 2 out]
      n443 = property on="実測設定項目配列_\nメインからの転記" class="Arr (指定)"() -> ("Value"=w1941:T1[])  [unwired: 2 in, 2 out]
      n444 = property on="実測設定項目配列_\nメインからの転記" class="Arr (指定)"() -> ("Value"=w1898:T1[])  [unwired: 2 in, 2 out]
      n445 = property on="実測設定項目配列_\nメインからの転記" class="Arr (指定)"() -> ("Value"=w1972:T1[])  [unwired: 2 in, 2 out]
      n446 = property on="実測設定項目配列_\nメインからの転記" class="Arr (指定)"() -> ("Value"=w1905:T1[])  [unwired: 2 in, 2 out]
      n447 = property on="実測設定項目配列_\nメインからの転記" class="Arr (指定)"() -> ("Value"=w1991:T1[])  [unwired: 2 in, 2 out]
      n448 = property on="実測設定項目配列_\nメインからの転記" class="Arr (指定)"() -> ("Value"=w1975:T1[])  [unwired: 2 in, 2 out]
      n449 = Index Array(array=w1934, index=w1937) -> (element=w1933:T1)
      n450 = Index Array(array=w1923, index=w1920) -> (element=w1924:T1)
      n451 = Index Array(array=w1916, index=w1919) -> (element=w1915:T1)
      n452 = Index Array(array=w1887, index=w1884) -> (element=w1888:T1)
      n453 = Index Array(array=w1959, index=w1956) -> (element=w1960:T1)
      n454 = Index Array(array=w1952, index=w1955) -> (element=w1951:T1)
      n455 = Index Array(array=w1941, index=w1938) -> (element=w1942:T1)
      n456 = Index Array(array=w1898, index=w1901) -> (element=w1897:T1)
      n457 = Index Array(array=w1972, index=w1965) -> (element=w1971:T1)
      n458 = Index Array(array=w1905, index=w1902) -> (element=w1906:T1)
      n459 = Index Array(array=w1991, index=w1981) -> (element=w1990:T1)
      n460 = Index Array(array=w1975, index=w1973) -> (element=w1976:T1)
      n461 = Unbundle By Name(w1933) -> ("ゲージポートNo"=w1930:refnum<visa-resource-name>)
      n462 = Unbundle By Name(w1924) -> ("ゲージポートNo"=w1927:refnum<visa-resource-name>)
      n463 = Unbundle By Name(w1915) -> ("ゲージポートNo"=w1912:refnum<visa-resource-name>)
      n464 = Unbundle By Name(w1888) -> ("ゲージポートNo"=w1891:refnum<visa-resource-name>)
      n465 = Unbundle By Name(w1960) -> ("ゲージポートNo"=w1963:refnum<visa-resource-name>)
      n466 = Unbundle By Name(w1951) -> ("ゲージポートNo"=w1948:refnum<visa-resource-name>)
      n467 = Unbundle By Name(w1942) -> ("ゲージポートNo"=w1945:refnum<visa-resource-name>)
      n468 = Unbundle By Name(w1897) -> ("ゲージポートNo"=w1894:refnum<visa-resource-name>)
      n469 = Unbundle By Name(w1971) -> ("ゲージポートNo"=w1968:refnum<visa-resource-name>)
      n470 = Unbundle By Name(w1906) -> ("ゲージポートNo"=w1909:refnum<visa-resource-name>)
      n471 = Unbundle By Name(w1990) -> ("ゲージポートNo"=w1984:refnum<visa-resource-name>)
      n472 = Unbundle By Name(w1976) -> ("ゲージポートNo"=w1979:refnum<visa-resource-name>)
      n473 = Empty String/Path?(string/path=w1930) -> (empty?=w1929:bool)
      n474 = Empty String/Path?(string/path=w1927) -> (empty?=w1928:bool)
      n475 = Empty String/Path?(string/path=w1912) -> (empty?=w1911:bool)
      n476 = Empty String/Path?(string/path=w1891) -> (empty?=w1892:bool)
      n477 = Empty String/Path?(string/path=w1963) -> (empty?=w1964:bool)
      n478 = Empty String/Path?(string/path=w1948) -> (empty?=w1947:bool)
      n479 = Empty String/Path?(string/path=w1945) -> (empty?=w1946:bool)
      n480 = Empty String/Path?(string/path=w1894) -> (empty?=w1893:bool)
      n481 = Empty String/Path?(string/path=w1968) -> (empty?=w1967:bool)
      n482 = Empty String/Path?(string/path=w1909) -> (empty?=w1910:bool)
      n483 = Empty String/Path?(string/path=w1984) -> (empty?=w1983:bool)
      n484 = Empty String/Path?(string/path=w1979) -> (empty?=w1980:bool)
      n485 = case shown="TRUE" w1929 {
        tunnel: [w2127 _] -> w1931
        tunnel: w1930 -> [w2130 _]
        tunnel: w1937 -> [_ w2135]
        tunnel: w1937 -> [_ w2134]
        tunnel: w1937 -> [_ w2133]
        frame False {
          n486 = VISA Open(VISA resource name=w2130) -> (VISA resource name=w2128:refnum<visa-resource-name>, error out=w2129:errorcluster)  [unwired: 4 in]
          n487 = case shown="エラーなし" w2129 {
            tunnel: w2128 -> [w2131 w2132]
            tunnel: [w2131 _] -> w2127
            frame No Error {
            }
            frame Error {
              n488 = VISA Close(VISA resource name=w2132) -> ()  [unwired: 1 in, 1 out]
            }
          }
        }
        frame True {
          n489 = for {
            N: 1 -> [_]
            tunnel: w2135 -> [w2139]
            tunnel: w2134 -> [w2138]
            tunnel: w2133 -> [w2137]
            i -> [w2140]
            n490 = case shown="0, デフォルト" w2140 {
              tunnel: w2139 -> [w2142 _]
              tunnel: w2138 -> [w2141 _]
              tunnel: w2137 -> [_ w2150]
              frame 0, Default {
                n491 = flat-sequence {
                  tunnel: w2142 -> [w2143]
                  tunnel: w2141 -> [w2146]
                  frame #0 {
                    n492 = global read "測定データ転記.vi" "測定転記一時データ"() -> (w2144:string[])
                    n493 = Delete From Array(array=w2144, index=w2143) -> (array with subset deleted=w2145:string[])  [unwired: 1 in, 1 out]
                    n494 = global write "測定データ転記.vi" "測定転記一時データ"(w2145) -> ()
                  }
                  frame #1 {
                    n495 = global read "測定データ転記.vi" "測定転記一時データ"() -> (w2149:string[])
                    n496 = Insert Into Array(array=w2149, index=w2146, new element="") -> (w2148:string[])
                    n497 = global write "測定データ転記.vi" "測定転記一時データ"(w2148) -> ()
                  }
                }
              }
              frame 1.. {
                n498 = global read "測定データ転記.vi" "測定転記一時データ"() -> (w2153:string[])
                n499 = Replace Array Subset(array=w2153, new element="", index=w2150) -> (w2152:string[])
                n500 = global write "測定データ転記.vi" "測定転記一時データ"(w2152) -> ()
              }
            }
          }
        }
      }
      n501 = case shown="TRUE" w1928 {
        tunnel: [w2100 _] -> w1926
        tunnel: w1927 -> [w2103 _]
        tunnel: w1920 -> [_ w2108]
        tunnel: w1920 -> [_ w2107]
        tunnel: w1920 -> [_ w2106]
        frame False {
          n502 = VISA Open(VISA resource name=w2103) -> (VISA resource name=w2101:refnum<visa-resource-name>, error out=w2102:errorcluster)  [unwired: 4 in]
          n503 = case shown="エラーなし" w2102 {
            tunnel: w2101 -> [w2104 w2105]
            tunnel: [w2104 _] -> w2100
            frame No Error {
            }
            frame Error {
              n504 = VISA Close(VISA resource name=w2105) -> ()  [unwired: 1 in, 1 out]
            }
          }
        }
        frame True {
          n505 = for {
            N: 1 -> [_]
            tunnel: w2108 -> [w2112]
            tunnel: w2107 -> [w2111]
            tunnel: w2106 -> [w2110]
            i -> [w2113]
            n506 = case shown="0, デフォルト" w2113 {
              tunnel: w2112 -> [w2115 _]
              tunnel: w2111 -> [w2114 _]
              tunnel: w2110 -> [_ w2123]
              frame 0, Default {
                n507 = flat-sequence {
                  tunnel: w2115 -> [w2116]
                  tunnel: w2114 -> [w2119]
                  frame #0 {
                    n508 = global read "測定データ転記.vi" "測定転記一時データ"() -> (w2117:string[])
                    n509 = Delete From Array(array=w2117, index=w2116) -> (array with subset deleted=w2118:string[])  [unwired: 1 in, 1 out]
                    n510 = global write "測定データ転記.vi" "測定転記一時データ"(w2118) -> ()
                  }
                  frame #1 {
                    n511 = global read "測定データ転記.vi" "測定転記一時データ"() -> (w2122:string[])
                    n512 = Insert Into Array(array=w2122, index=w2119, new element="") -> (w2121:string[])
                    n513 = global write "測定データ転記.vi" "測定転記一時データ"(w2121) -> ()
                  }
                }
              }
              frame 1.. {
                n514 = global read "測定データ転記.vi" "測定転記一時データ"() -> (w2126:string[])
                n515 = Replace Array Subset(array=w2126, new element="", index=w2123) -> (w2125:string[])
                n516 = global write "測定データ転記.vi" "測定転記一時データ"(w2125) -> ()
              }
            }
          }
        }
      }
      n517 = case shown="TRUE" w1911 {
        tunnel: [w2073 _] -> w1913
        tunnel: w1912 -> [w2076 _]
        tunnel: w1919 -> [_ w2081]
        tunnel: w1919 -> [_ w2080]
        tunnel: w1919 -> [_ w2079]
        frame False {
          n518 = VISA Open(VISA resource name=w2076) -> (VISA resource name=w2074:refnum<visa-resource-name>, error out=w2075:errorcluster)  [unwired: 4 in]
          n519 = case shown="エラーなし" w2075 {
            tunnel: w2074 -> [w2077 w2078]
            tunnel: [w2077 _] -> w2073
            frame No Error {
            }
            frame Error {
              n520 = VISA Close(VISA resource name=w2078) -> ()  [unwired: 1 in, 1 out]
            }
          }
        }
        frame True {
          n521 = for {
            N: 1 -> [_]
            tunnel: w2081 -> [w2085]
            tunnel: w2080 -> [w2084]
            tunnel: w2079 -> [w2083]
            i -> [w2086]
            n522 = case shown="0, デフォルト" w2086 {
              tunnel: w2085 -> [w2088 _]
              tunnel: w2084 -> [w2087 _]
              tunnel: w2083 -> [_ w2096]
              frame 0, Default {
                n523 = flat-sequence {
                  tunnel: w2088 -> [w2089]
                  tunnel: w2087 -> [w2092]
                  frame #0 {
                    n524 = global read "測定データ転記.vi" "測定転記一時データ"() -> (w2090:string[])
                    n525 = Delete From Array(array=w2090, index=w2089) -> (array with subset deleted=w2091:string[])  [unwired: 1 in, 1 out]
                    n526 = global write "測定データ転記.vi" "測定転記一時データ"(w2091) -> ()
                  }
                  frame #1 {
                    n527 = global read "測定データ転記.vi" "測定転記一時データ"() -> (w2095:string[])
                    n528 = Insert Into Array(array=w2095, index=w2092, new element="") -> (w2094:string[])
                    n529 = global write "測定データ転記.vi" "測定転記一時データ"(w2094) -> ()
                  }
                }
              }
              frame 1.. {
                n530 = global read "測定データ転記.vi" "測定転記一時データ"() -> (w2099:string[])
                n531 = Replace Array Subset(array=w2099, new element="", index=w2096) -> (w2098:string[])
                n532 = global write "測定データ転記.vi" "測定転記一時データ"(w2098) -> ()
              }
            }
          }
        }
      }
      n533 = case shown="TRUE" w1892 {
        tunnel: [w1992 _] -> w1890
        tunnel: w1891 -> [w1995 _]
        tunnel: w1884 -> [_ w2000]
        tunnel: w1884 -> [_ w1999]
        tunnel: w1884 -> [_ w1998]
        frame False {
          n534 = VISA Open(VISA resource name=w1995) -> (VISA resource name=w1993:refnum<visa-resource-name>, error out=w1994:errorcluster)  [unwired: 4 in]
          n535 = case shown="エラーなし" w1994 {
            tunnel: w1993 -> [w1996 w1997]
            tunnel: [w1996 _] -> w1992
            frame No Error {
            }
            frame Error {
              n536 = VISA Close(VISA resource name=w1997) -> ()  [unwired: 1 in, 1 out]
            }
          }
        }
        frame True {
          n537 = for {
            N: 1 -> [_]
            tunnel: w2000 -> [w2004]
            tunnel: w1999 -> [w2003]
            tunnel: w1998 -> [w2002]
            i -> [w2005]
            n538 = case shown="0, デフォルト" w2005 {
              tunnel: w2004 -> [w2007 _]
              tunnel: w2003 -> [w2006 _]
              tunnel: w2002 -> [_ w2015]
              frame 0, Default {
                n539 = flat-sequence {
                  tunnel: w2007 -> [w2008]
                  tunnel: w2006 -> [w2011]
                  frame #0 {
                    n540 = global read "測定データ転記.vi" "測定転記一時データ"() -> (w2009:string[])
                    n541 = Delete From Array(array=w2009, index=w2008) -> (array with subset deleted=w2010:string[])  [unwired: 1 in, 1 out]
                    n542 = global write "測定データ転記.vi" "測定転記一時データ"(w2010) -> ()
                  }
                  frame #1 {
                    n543 = global read "測定データ転記.vi" "測定転記一時データ"() -> (w2014:string[])
                    n544 = Insert Into Array(array=w2014, index=w2011, new element="") -> (w2013:string[])
                    n545 = global write "測定データ転記.vi" "測定転記一時データ"(w2013) -> ()
                  }
                }
              }
              frame 1.. {
                n546 = global read "測定データ転記.vi" "測定転記一時データ"() -> (w2018:string[])
                n547 = Replace Array Subset(array=w2018, new element="", index=w2015) -> (w2017:string[])
                n548 = global write "測定データ転記.vi" "測定転記一時データ"(w2017) -> ()
              }
            }
          }
        }
      }
      n549 = case shown="TRUE" w1964 {
        tunnel: [w2208 _] -> w1962
        tunnel: w1963 -> [w2211 _]
        tunnel: w1956 -> [_ w2216]
        tunnel: w1956 -> [_ w2215]
        tunnel: w1956 -> [_ w2214]
        frame False {
          n550 = VISA Open(VISA resource name=w2211) -> (VISA resource name=w2209:refnum<visa-resource-name>, error out=w2210:errorcluster)  [unwired: 4 in]
          n551 = case shown="エラーなし" w2210 {
            tunnel: w2209 -> [w2212 w2213]
            tunnel: [w2212 _] -> w2208
            frame No Error {
            }
            frame Error {
              n552 = VISA Close(VISA resource name=w2213) -> ()  [unwired: 1 in, 1 out]
            }
          }
        }
        frame True {
          n553 = for {
            N: 1 -> [_]
            tunnel: w2216 -> [w2220]
            tunnel: w2215 -> [w2219]
            tunnel: w2214 -> [w2218]
            i -> [w2221]
            n554 = case shown="0, デフォルト" w2221 {
              tunnel: w2220 -> [w2223 _]
              tunnel: w2219 -> [w2222 _]
              tunnel: w2218 -> [_ w2231]
              frame 0, Default {
                n555 = flat-sequence {
                  tunnel: w2223 -> [w2224]
                  tunnel: w2222 -> [w2227]
                  frame #0 {
                    n556 = global read "測定データ転記.vi" "測定転記一時データ"() -> (w2225:string[])
                    n557 = Delete From Array(array=w2225, index=w2224) -> (array with subset deleted=w2226:string[])  [unwired: 1 in, 1 out]
                    n558 = global write "測定データ転記.vi" "測定転記一時データ"(w2226) -> ()
                  }
                  frame #1 {
                    n559 = global read "測定データ転記.vi" "測定転記一時データ"() -> (w2230:string[])
                    n560 = Insert Into Array(array=w2230, index=w2227, new element="") -> (w2229:string[])
                    n561 = global write "測定データ転記.vi" "測定転記一時データ"(w2229) -> ()
                  }
                }
              }
              frame 1.. {
                n562 = global read "測定データ転記.vi" "測定転記一時データ"() -> (w2234:string[])
                n563 = Replace Array Subset(array=w2234, new element="", index=w2231) -> (w2233:string[])
                n564 = global write "測定データ転記.vi" "測定転記一時データ"(w2233) -> ()
              }
            }
          }
        }
      }
      n565 = case shown="TRUE" w1947 {
        tunnel: [w2181 _] -> w1949
        tunnel: w1948 -> [w2184 _]
        tunnel: w1955 -> [_ w2189]
        tunnel: w1955 -> [_ w2188]
        tunnel: w1955 -> [_ w2187]
        frame False {
          n566 = VISA Open(VISA resource name=w2184) -> (VISA resource name=w2182:refnum<visa-resource-name>, error out=w2183:errorcluster)  [unwired: 4 in]
          n567 = case shown="エラーなし" w2183 {
            tunnel: w2182 -> [w2185 w2186]
            tunnel: [w2185 _] -> w2181
            frame No Error {
            }
            frame Error {
              n568 = VISA Close(VISA resource name=w2186) -> ()  [unwired: 1 in, 1 out]
            }
          }
        }
        frame True {
          n569 = for {
            N: 1 -> [_]
            tunnel: w2189 -> [w2193]
            tunnel: w2188 -> [w2192]
            tunnel: w2187 -> [w2191]
            i -> [w2194]
            n570 = case shown="0, デフォルト" w2194 {
              tunnel: w2193 -> [w2196 _]
              tunnel: w2192 -> [w2195 _]
              tunnel: w2191 -> [_ w2204]
              frame 0, Default {
                n571 = flat-sequence {
                  tunnel: w2196 -> [w2197]
                  tunnel: w2195 -> [w2200]
                  frame #0 {
                    n572 = global read "測定データ転記.vi" "測定転記一時データ"() -> (w2198:string[])
                    n573 = Delete From Array(array=w2198, index=w2197) -> (array with subset deleted=w2199:string[])  [unwired: 1 in, 1 out]
                    n574 = global write "測定データ転記.vi" "測定転記一時データ"(w2199) -> ()
                  }
                  frame #1 {
                    n575 = global read "測定データ転記.vi" "測定転記一時データ"() -> (w2203:string[])
                    n576 = Insert Into Array(array=w2203, index=w2200, new element="") -> (w2202:string[])
                    n577 = global write "測定データ転記.vi" "測定転記一時データ"(w2202) -> ()
                  }
                }
              }
              frame 1.. {
                n578 = global read "測定データ転記.vi" "測定転記一時データ"() -> (w2207:string[])
                n579 = Replace Array Subset(array=w2207, new element="", index=w2204) -> (w2206:string[])
                n580 = global write "測定データ転記.vi" "測定転記一時データ"(w2206) -> ()
              }
            }
          }
        }
      }
      n581 = case shown="TRUE" w1946 {
        tunnel: [w2154 _] -> w1944
        tunnel: w1945 -> [w2157 _]
        tunnel: w1938 -> [_ w2162]
        tunnel: w1938 -> [_ w2161]
        tunnel: w1938 -> [_ w2160]
        frame False {
          n582 = VISA Open(VISA resource name=w2157) -> (VISA resource name=w2155:refnum<visa-resource-name>, error out=w2156:errorcluster)  [unwired: 4 in]
          n583 = case shown="エラーなし" w2156 {
            tunnel: w2155 -> [w2158 w2159]
            tunnel: [w2158 _] -> w2154
            frame No Error {
            }
            frame Error {
              n584 = VISA Close(VISA resource name=w2159) -> ()  [unwired: 1 in, 1 out]
            }
          }
        }
        frame True {
          n585 = for {
            N: 1 -> [_]
            tunnel: w2162 -> [w2166]
            tunnel: w2161 -> [w2165]
            tunnel: w2160 -> [w2164]
            i -> [w2167]
            n586 = case shown="0, デフォルト" w2167 {
              tunnel: w2166 -> [w2169 _]
              tunnel: w2165 -> [w2168 _]
              tunnel: w2164 -> [_ w2177]
              frame 0, Default {
                n587 = flat-sequence {
                  tunnel: w2169 -> [w2170]
                  tunnel: w2168 -> [w2173]
                  frame #0 {
                    n588 = global read "測定データ転記.vi" "測定転記一時データ"() -> (w2171:string[])
                    n589 = Delete From Array(array=w2171, index=w2170) -> (array with subset deleted=w2172:string[])  [unwired: 1 in, 1 out]
                    n590 = global write "測定データ転記.vi" "測定転記一時データ"(w2172) -> ()
                  }
                  frame #1 {
                    n591 = global read "測定データ転記.vi" "測定転記一時データ"() -> (w2176:string[])
                    n592 = Insert Into Array(array=w2176, index=w2173, new element="") -> (w2175:string[])
                    n593 = global write "測定データ転記.vi" "測定転記一時データ"(w2175) -> ()
                  }
                }
              }
              frame 1.. {
                n594 = global read "測定データ転記.vi" "測定転記一時データ"() -> (w2180:string[])
                n595 = Replace Array Subset(array=w2180, new element="", index=w2177) -> (w2179:string[])
                n596 = global write "測定データ転記.vi" "測定転記一時データ"(w2179) -> ()
              }
            }
          }
        }
      }
      n597 = case shown="TRUE" w1893 {
        tunnel: [w2019 _] -> w1895
        tunnel: w1894 -> [w2022 _]
        tunnel: w1901 -> [_ w2027]
        tunnel: w1901 -> [_ w2026]
        tunnel: w1901 -> [_ w2025]
        frame False {
          n598 = VISA Open(VISA resource name=w2022) -> (VISA resource name=w2020:refnum<visa-resource-name>, error out=w2021:errorcluster)  [unwired: 4 in]
          n599 = case shown="エラーなし" w2021 {
            tunnel: w2020 -> [w2023 w2024]
            tunnel: [w2023 _] -> w2019
            frame No Error {
            }
            frame Error {
              n600 = VISA Close(VISA resource name=w2024) -> ()  [unwired: 1 in, 1 out]
            }
          }
        }
        frame True {
          n601 = for {
            N: 1 -> [_]
            tunnel: w2027 -> [w2031]
            tunnel: w2026 -> [w2030]
            tunnel: w2025 -> [w2029]
            i -> [w2032]
            n602 = case shown="0, デフォルト" w2032 {
              tunnel: w2031 -> [w2034 _]
              tunnel: w2030 -> [w2033 _]
              tunnel: w2029 -> [_ w2042]
              frame 0, Default {
                n603 = flat-sequence {
                  tunnel: w2034 -> [w2035]
                  tunnel: w2033 -> [w2038]
                  frame #0 {
                    n604 = global read "測定データ転記.vi" "測定転記一時データ"() -> (w2036:string[])
                    n605 = Delete From Array(array=w2036, index=w2035) -> (array with subset deleted=w2037:string[])  [unwired: 1 in, 1 out]
                    n606 = global write "測定データ転記.vi" "測定転記一時データ"(w2037) -> ()
                  }
                  frame #1 {
                    n607 = global read "測定データ転記.vi" "測定転記一時データ"() -> (w2041:string[])
                    n608 = Insert Into Array(array=w2041, index=w2038, new element="") -> (w2040:string[])
                    n609 = global write "測定データ転記.vi" "測定転記一時データ"(w2040) -> ()
                  }
                }
              }
              frame 1.. {
                n610 = global read "測定データ転記.vi" "測定転記一時データ"() -> (w2045:string[])
                n611 = Replace Array Subset(array=w2045, new element="", index=w2042) -> (w2044:string[])
                n612 = global write "測定データ転記.vi" "測定転記一時データ"(w2044) -> ()
              }
            }
          }
        }
      }
      n613 = case shown="TRUE" w1967 {
        tunnel: [w2235 _] -> w1969
        tunnel: w1968 -> [w2238 _]
        tunnel: w1965 -> [_ w2243]
        tunnel: w1965 -> [_ w2242]
        tunnel: w1965 -> [_ w2241]
        frame False {
          n614 = VISA Open(VISA resource name=w2238) -> (VISA resource name=w2236:refnum<visa-resource-name>, error out=w2237:errorcluster)  [unwired: 4 in]
          n615 = case shown="エラーなし" w2237 {
            tunnel: w2236 -> [w2239 w2240]
            tunnel: [w2239 _] -> w2235
            frame No Error {
            }
            frame Error {
              n616 = VISA Close(VISA resource name=w2240) -> ()  [unwired: 1 in, 1 out]
            }
          }
        }
        frame True {
          n617 = for {
            N: 1 -> [_]
            tunnel: w2243 -> [w2247]
            tunnel: w2242 -> [w2246]
            tunnel: w2241 -> [w2245]
            i -> [w2248]
            n618 = case shown="0, デフォルト" w2248 {
              tunnel: w2247 -> [w2250 _]
              tunnel: w2246 -> [w2249 _]
              tunnel: w2245 -> [_ w2258]
              frame 0, Default {
                n619 = flat-sequence {
                  tunnel: w2250 -> [w2251]
                  tunnel: w2249 -> [w2254]
                  frame #0 {
                    n620 = global read "測定データ転記.vi" "測定転記一時データ"() -> (w2252:string[])
                    n621 = Delete From Array(array=w2252, index=w2251) -> (array with subset deleted=w2253:string[])  [unwired: 1 in, 1 out]
                    n622 = global write "測定データ転記.vi" "測定転記一時データ"(w2253) -> ()
                  }
                  frame #1 {
                    n623 = global read "測定データ転記.vi" "測定転記一時データ"() -> (w2257:string[])
                    n624 = Insert Into Array(array=w2257, index=w2254, new element="") -> (w2256:string[])
                    n625 = global write "測定データ転記.vi" "測定転記一時データ"(w2256) -> ()
                  }
                }
              }
              frame 1.. {
                n626 = global read "測定データ転記.vi" "測定転記一時データ"() -> (w2261:string[])
                n627 = Replace Array Subset(array=w2261, new element="", index=w2258) -> (w2260:string[])
                n628 = global write "測定データ転記.vi" "測定転記一時データ"(w2260) -> ()
              }
            }
          }
        }
      }
      n629 = case shown="TRUE" w1910 {
        tunnel: [w2046 _] -> w1908
        tunnel: w1909 -> [w2049 _]
        tunnel: w1902 -> [_ w2054]
        tunnel: w1902 -> [_ w2053]
        tunnel: w1902 -> [_ w2052]
        frame False {
          n630 = VISA Open(VISA resource name=w2049) -> (VISA resource name=w2047:refnum<visa-resource-name>, error out=w2048:errorcluster)  [unwired: 4 in]
          n631 = case shown="エラーなし" w2048 {
            tunnel: w2047 -> [w2050 w2051]
            tunnel: [w2050 _] -> w2046
            frame No Error {
            }
            frame Error {
              n632 = VISA Close(VISA resource name=w2051) -> ()  [unwired: 1 in, 1 out]
            }
          }
        }
        frame True {
          n633 = for {
            N: 1 -> [_]
            tunnel: w2054 -> [w2058]
            tunnel: w2053 -> [w2057]
            tunnel: w2052 -> [w2056]
            i -> [w2059]
            n634 = case shown="0, デフォルト" w2059 {
              tunnel: w2058 -> [w2061 _]
              tunnel: w2057 -> [w2060 _]
              tunnel: w2056 -> [_ w2069]
              frame 0, Default {
                n635 = flat-sequence {
                  tunnel: w2061 -> [w2062]
                  tunnel: w2060 -> [w2065]
                  frame #0 {
                    n636 = global read "測定データ転記.vi" "測定転記一時データ"() -> (w2063:string[])
                    n637 = Delete From Array(array=w2063, index=w2062) -> (array with subset deleted=w2064:string[])  [unwired: 1 in, 1 out]
                    n638 = global write "測定データ転記.vi" "測定転記一時データ"(w2064) -> ()
                  }
                  frame #1 {
                    n639 = global read "測定データ転記.vi" "測定転記一時データ"() -> (w2068:string[])
                    n640 = Insert Into Array(array=w2068, index=w2065, new element="") -> (w2067:string[])
                    n641 = global write "測定データ転記.vi" "測定転記一時データ"(w2067) -> ()
                  }
                }
              }
              frame 1.. {
                n642 = global read "測定データ転記.vi" "測定転記一時データ"() -> (w2072:string[])
                n643 = Replace Array Subset(array=w2072, new element="", index=w2069) -> (w2071:string[])
                n644 = global write "測定データ転記.vi" "測定転記一時データ"(w2071) -> ()
              }
            }
          }
        }
      }
      n645 = case shown="TRUE" w1983 {
        tunnel: [w2346 _] -> w1987
        tunnel: w1984 -> [w2349 _]
        tunnel: w1981 -> [_ w2354]
        tunnel: w1981 -> [_ w2353]
        tunnel: w1981 -> [_ w2352]
        frame False {
          n646 = VISA Open(VISA resource name=w2349) -> (VISA resource name=w2347:refnum<visa-resource-name>, error out=w2348:errorcluster)  [unwired: 4 in]
          n647 = case shown="エラーなし" w2348 {
            tunnel: w2347 -> [w2350 w2351]
            tunnel: [w2350 _] -> w2346
            frame No Error {
            }
            frame Error {
              n648 = VISA Close(VISA resource name=w2351) -> ()  [unwired: 1 in, 1 out]
            }
          }
        }
        frame True {
          n649 = for {
            N: 1 -> [_]
            tunnel: w2354 -> [w2358]
            tunnel: w2353 -> [w2357]
            tunnel: w2352 -> [w2356]
            i -> [w2359]
            n650 = case shown="0, デフォルト" w2359 {
              tunnel: w2358 -> [w2361 _]
              tunnel: w2357 -> [w2360 _]
              tunnel: w2356 -> [_ w2369]
              frame 0, Default {
                n651 = flat-sequence {
                  tunnel: w2361 -> [w2362]
                  tunnel: w2360 -> [w2365]
                  frame #0 {
                    n652 = global read "測定データ転記.vi" "測定転記一時データ"() -> (w2363:string[])
                    n653 = Delete From Array(array=w2363, index=w2362) -> (array with subset deleted=w2364:string[])  [unwired: 1 in, 1 out]
                    n654 = global write "測定データ転記.vi" "測定転記一時データ"(w2364) -> ()
                  }
                  frame #1 {
                    n655 = global read "測定データ転記.vi" "測定転記一時データ"() -> (w2368:string[])
                    n656 = Insert Into Array(array=w2368, index=w2365, new element="") -> (w2367:string[])
                    n657 = global write "測定データ転記.vi" "測定転記一時データ"(w2367) -> ()
                  }
                }
              }
              frame 1.. {
                n658 = global read "測定データ転記.vi" "測定転記一時データ"() -> (w2372:string[])
                n659 = Replace Array Subset(array=w2372, new element="", index=w2369) -> (w2371:string[])
                n660 = global write "測定データ転記.vi" "測定転記一時データ"(w2371) -> ()
              }
            }
          }
        }
      }
      n661 = case shown="TRUE" w1980 {
        tunnel: [w2262 _] -> w1978
        tunnel: w1979 -> [w2265 _]
        tunnel: w1973 -> [_ w2270]
        tunnel: w1973 -> [_ w2269]
        tunnel: w1973 -> [_ w2268]
        frame False {
          n662 = VISA Open(VISA resource name=w2265) -> (VISA resource name=w2263:refnum<visa-resource-name>, error out=w2264:errorcluster)  [unwired: 4 in]
          n663 = case shown="エラーなし" w2264 {
            tunnel: w2263 -> [w2266 w2267]
            tunnel: [w2266 _] -> w2262
            frame No Error {
            }
            frame Error {
              n664 = VISA Close(VISA resource name=w2267) -> ()  [unwired: 1 in, 1 out]
            }
          }
        }
        frame True {
          n665 = for {
            N: 1 -> [_]
            tunnel: w2270 -> [w2274]
            tunnel: w2269 -> [w2273]
            tunnel: w2268 -> [w2272]
            i -> [w2275]
            n666 = case shown="0, デフォルト" w2275 {
              tunnel: w2274 -> [w2277 _]
              tunnel: w2273 -> [w2276 _]
              tunnel: w2272 -> [_ w2285]
              frame 0, Default {
                n667 = flat-sequence {
                  tunnel: w2277 -> [w2278]
                  tunnel: w2276 -> [w2281]
                  frame #0 {
                    n668 = global read "測定データ転記.vi" "測定転記一時データ"() -> (w2279:string[])
                    n669 = Delete From Array(array=w2279, index=w2278) -> (array with subset deleted=w2280:string[])  [unwired: 1 in, 1 out]
                    n670 = global write "測定データ転記.vi" "測定転記一時データ"(w2280) -> ()
                  }
                  frame #1 {
                    n671 = global read "測定データ転記.vi" "測定転記一時データ"() -> (w2284:string[])
                    n672 = Insert Into Array(array=w2284, index=w2281, new element="") -> (w2283:string[])
                    n673 = global write "測定データ転記.vi" "測定転記一時データ"(w2283) -> ()
                  }
                }
              }
              frame 1.. {
                n674 = global read "測定データ転記.vi" "測定転記一時データ"() -> (w2288:string[])
                n675 = Replace Array Subset(array=w2288, new element="", index=w2285) -> (w2287:string[])
                n676 = global write "測定データ転記.vi" "測定転記一時データ"(w2287) -> ()
              }
            }
          }
        }
      }
      n677 = property class="Instr"(reference=w1931, "TermChar"=u8 13 ("Message Based Settings:Termination Character")) -> (reference out=w1936:refnum<visa-resource-name>)  [unwired: 1 in, 1 out]
      n678 = property class="Instr"(reference=w1926, "TermChar"=u8 13 ("Message Based Settings:Termination Character")) -> (reference out=w1921:refnum<visa-resource-name>)  [unwired: 1 in, 1 out]
      n679 = property class="Instr"(reference=w1913, "TermChar"=u8 13 ("Message Based Settings:Termination Character")) -> (reference out=w1918:refnum<visa-resource-name>)  [unwired: 1 in, 1 out]
      n680 = property class="Instr"(reference=w1890, "TermChar"=u8 13 ("Message Based Settings:Termination Character")) -> (reference out=w1885:refnum<visa-resource-name>)  [unwired: 1 in, 1 out]
      n681 = property class="Instr"(reference=w1962, "TermChar"=u8 13 ("Message Based Settings:Termination Character")) -> (reference out=w1957:refnum<visa-resource-name>)  [unwired: 1 in, 1 out]
      n682 = property class="Instr"(reference=w1949, "TermChar"=u8 13 ("Message Based Settings:Termination Character")) -> (reference out=w1954:refnum<visa-resource-name>)  [unwired: 1 in, 1 out]
      n683 = property class="Instr"(reference=w1944, "TermChar"=u8 13 ("Message Based Settings:Termination Character")) -> (reference out=w1939:refnum<visa-resource-name>)  [unwired: 1 in, 1 out]
      n684 = property class="Instr"(reference=w1895, "TermChar"=u8 13 ("Message Based Settings:Termination Character")) -> (reference out=w1900:refnum<visa-resource-name>)  [unwired: 1 in, 1 out]
      n685 = property class="Instr"(reference=w1969, "TermChar"=u8 13 ("Message Based Settings:Termination Character")) -> (reference out=w1966:refnum<visa-resource-name>)  [unwired: 1 in, 1 out]
      n686 = property class="Instr"(reference=w1908, "TermChar"=u8 13 ("Message Based Settings:Termination Character")) -> (reference out=w1903:refnum<visa-resource-name>)  [unwired: 1 in, 1 out]
      n687 = property class="Instr"(reference=w1987, "TermChar"=u8 13 ("Message Based Settings:Termination Character")) -> (reference out=w1989:refnum<visa-resource-name>)  [unwired: 1 in, 1 out]
      n688 = property class="Instr"(reference=w1978, "TermChar"=u8 13 ("Message Based Settings:Termination Character")) -> (reference out=w1974:refnum<visa-resource-name>)  [unwired: 1 in, 1 out]
      n689 = while {
        tunnel: w1989 -> [w2338]
        tunnel: w1974 -> [w2336]
        tunnel: [w2337] -> w1986
        tunnel: w1966 -> [w2333]
        tunnel: [w2334] -> w1985
        tunnel: w1982 -> [w2331]
        tunnel: w1981 -> [w2330]
        tunnel: w1973 -> [w2329]
        tunnel: w1965 -> [w2328]
        tunnel: [w2326] -> w1958
        tunnel: w1957 -> [w2325]
        tunnel: w1956 -> [w2324]
        tunnel: [w2321] -> w1953
        tunnel: w1954 -> [w2322]
        tunnel: w1955 -> [w2323]
        tunnel: [w2318] -> w1940
        tunnel: w1939 -> [w2317]
        tunnel: w1938 -> [w2316]
        tunnel: [w2313] -> w1935
        tunnel: w1936 -> [w2314]
        tunnel: w1937 -> [w2315]
        tunnel: [w2310] -> w1922
        tunnel: w1921 -> [w2309]
        tunnel: w1920 -> [w2308]
        tunnel: [w2305] -> w1917
        tunnel: w1918 -> [w2306]
        tunnel: w1919 -> [w2307]
        tunnel: [w2302] -> w1904
        tunnel: w1903 -> [w2301]
        tunnel: w1902 -> [w2300]
        tunnel: [w2297] -> w1899
        tunnel: w1900 -> [w2298]
        tunnel: w1901 -> [w2299]
        tunnel: [w2294] -> w1886
        tunnel: w1885 -> [w2293]
        tunnel: w1884 -> [w2292]
        i -> [w2291]
        stop <- w2290 stop-if-true
        n690 = stacked-sequence {
          tunnel: [w2342] -> w2289
          tunnel: w2330 -> [_]
          tunnel: w2291 -> [_]
          tunnel: w2338 -> [w2345]
          frame #0 {
            n691 = Concatenate Strings("P" ("書き込みバッファ"), "92" ("書き込みバッファ"), "\r") -> (w2343:string)
            n692 = VISA Write(VISA resource name=w2345, write buffer=w2343) -> (VISA resource name out=w2339:refnum<visa-resource-name>, error out=w2342:errorcluster)  [unwired: 1 in, 1 out]
            n693 = VISA Close(VISA resource name=w2339) -> ()  [unwired: 1 in, 1 out]
          }
        }
        "ゲージエラー 1" <- w2289
        n694 = call "ゲージデータ取り込み_サブ1.vi"("配列指標"=w2329, "ループ回数数値"=w2291, "VISA Refnum入力"=w2336) -> ("エラー出力"=→"ゲージエラー 2":errorcluster, "VISA Refnum出力"=w2337:refnum<visa-resource-name>)  [unwired: 7 in]
        n695 = call "ゲージデータ取り込み_サブ1.vi"("配列指標"=w2315, "ループ回数数値"=w2291, "VISA Refnum入力"=w2314) -> ("エラー出力"=→"ゲージエラー 7":errorcluster, "VISA Refnum出力"=w2313:refnum<visa-resource-name>)  [unwired: 7 in]
        n696 = call "ゲージデータ取り込み_サブ1.vi"("配列指標"=w2308, "ループ回数数値"=w2291, "VISA Refnum入力"=w2309) -> ("エラー出力"=→"ゲージエラー 8":errorcluster, "VISA Refnum出力"=w2310:refnum<visa-resource-name>)  [unwired: 7 in]
        n697 = call "ゲージデータ取り込み_サブ1.vi"("配列指標"=w2307, "ループ回数数値"=w2291, "VISA Refnum入力"=w2306) -> ("エラー出力"=→"ゲージエラー 9":errorcluster, "VISA Refnum出力"=w2305:refnum<visa-resource-name>)  [unwired: 7 in]
        n698 = call "ゲージデータ取り込み_サブ1.vi"("配列指標"=w2292, "ループ回数数値"=w2291, "VISA Refnum入力"=w2293) -> ("エラー出力"=→"ゲージエラー 12":errorcluster, "VISA Refnum出力"=w2294:refnum<visa-resource-name>)  [unwired: 7 in]
        n699 = call "ゲージデータ取り込み_サブ1.vi"("配列指標"=w2328, "ループ回数数値"=w2291, "VISA Refnum入力"=w2333) -> ("エラー出力"=→"ゲージエラー 3":errorcluster, "VISA Refnum出力"=w2334:refnum<visa-resource-name>)  [unwired: 7 in]
        n700 = call "ゲージデータ取り込み_サブ1.vi"("配列指標"=w2324, "ループ回数数値"=w2291, "VISA Refnum入力"=w2325) -> ("エラー出力"=→"ゲージエラー 4":errorcluster, "VISA Refnum出力"=w2326:refnum<visa-resource-name>)  [unwired: 7 in]
        n701 = call "ゲージデータ取り込み_サブ1.vi"("配列指標"=w2323, "ループ回数数値"=w2291, "VISA Refnum入力"=w2322) -> ("エラー出力"=→"ゲージエラー 5":errorcluster, "VISA Refnum出力"=w2321:refnum<visa-resource-name>)  [unwired: 7 in]
        n702 = call "ゲージデータ取り込み_サブ1.vi"("配列指標"=w2316, "ループ回数数値"=w2291, "VISA Refnum入力"=w2317) -> ("エラー出力"=→"ゲージエラー 6":errorcluster, "VISA Refnum出力"=w2318:refnum<visa-resource-name>)  [unwired: 7 in]
        n703 = call "ゲージデータ取り込み_サブ1.vi"("配列指標"=w2299, "ループ回数数値"=w2291, "VISA Refnum入力"=w2298) -> ("エラー出力"=→"ゲージエラー 11":errorcluster, "VISA Refnum出力"=w2297:refnum<visa-resource-name>)  [unwired: 7 in]
        n704 = call "ゲージデータ取り込み_サブ1.vi"("配列指標"=w2300, "ループ回数数値"=w2291, "VISA Refnum入力"=w2301) -> ("エラー出力"=→"ゲージエラー 10":errorcluster, "VISA Refnum出力"=w2302:refnum<visa-resource-name>)  [unwired: 7 in]
        n705 = Wait Until Next ms Multiple(millisecond multiple=w2331) -> ()  [unwired: 1 out]
        n706 = global read "VISA停止_G.vi" "VISA停止_\nグローバル"() -> (w2290:bool)
      }
      n707 = VISA Close(VISA resource name=w1935) -> ()  [unwired: 1 in, 1 out]
      n708 = VISA Close(VISA resource name=w1922) -> ()  [unwired: 1 in, 1 out]
      n709 = VISA Close(VISA resource name=w1917) -> ()  [unwired: 1 in, 1 out]
      n710 = VISA Close(VISA resource name=w1886) -> ()  [unwired: 1 in, 1 out]
      n711 = VISA Close(VISA resource name=w1986) -> ()  [unwired: 1 in, 1 out]
      n712 = VISA Close(VISA resource name=w1985) -> ()  [unwired: 1 in, 1 out]
      n713 = VISA Close(VISA resource name=w1958) -> ()  [unwired: 1 in, 1 out]
      n714 = VISA Close(VISA resource name=w1953) -> ()  [unwired: 1 in, 1 out]
      n715 = VISA Close(VISA resource name=w1940) -> ()  [unwired: 1 in, 1 out]
      n716 = VISA Close(VISA resource name=w1899) -> ()  [unwired: 1 in, 1 out]
      n717 = VISA Close(VISA resource name=w1904) -> ()  [unwired: 1 in, 1 out]
    }
  }
